vi "MM.vi"(0 "AppInst":refnum<vi>, 1 "ActorMethod":path, 2 "ActorClassItemRef(Don't Delete)":refnum<vi>, 3 "OnlyUpdate(if needed,False)":bool, 4 "Destination Path":path, 5 "error in":errorcluster, 6 "TemplatePath":path, 8 "TemplateVersion":string) -> (19 "error out":errorcluster)   [LabVIEW 2020]
uses:
  <vilib>/Utility/VariantDataType/Type.ctl
  <vilib>/Utility/miscctls.llb/LVPositionTypeDef.ctl
  <vilib>/Utility/traverseref.llb/TRef TravTarget.ctl
  <resource>/Framework/Providers/Open_GDS/ClassProviders/Common/LvClass_class/GDSLvCLass_ClassSettingsType.ctl
  <resource>/Framework/Providers/Open_GDS/ClassProviders/Common/LvClass_class/GDSLvClass_PlugIn.ctl
  <resource>/Framework/Providers/Open_GDS/ClassProviders/Common/LvClass_class/GDSLvClass_PlugInTypes.ctl
  <resource>/Framework/Providers/Open_GDS/ClassProviders/Provider_LvNativeClass/LvNativeProviderName.ctl
  <vilib>/Utility/VariantDataType/VariantType.lvlib
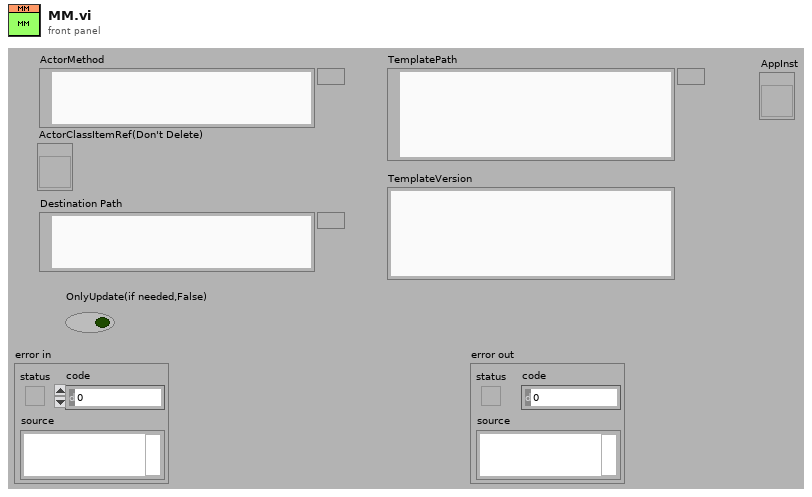
[diagram p1: front panel]
types:
  T1 = cluster{"Counter":i32, "DebugInfo":string, "Update":bool, "Target Actor Method path":path, "Class Name":string, "New Class Path":path, "Wiring Rules":enum16{"Invalid Wire Rule", "Required", "Recommended", "Optional", "Dynamic Dispatch"}[], "New Send Method":path, "Pattern":u32, "NewClassName":string, "NewClasstypeString":string, "Destination Path":path, "MessageClassRef":refnum<vi>, "Version":string, "ActorClassRef":refnum<vi>, "QualifiedNameOfLibrary":string, "TemplatePath":path, "ActorClassPath":path, "MemberDataTypes":cluster{"Label.Text":string, "Style":u32}[], "MemberData":refnum<vi>, "ActorClassParentItem":refnum<vi>}
  T2 = enum32{"Invalid", "Standard", "Closed", "Hidden", "Minimized", "Maximized"}
  T3 = typedef "LVPositionTypeDef.ctl" = cluster{"Left":i32, "Top":i32}
  T4 = typedef "TRef TravTarget.ctl" = enum16{"FP", "BD", "Other"}
  T5 = typedef "LvNativeProviderName.ctl" = enum16{"Endevo LabVIEW Native"}
  T6 = typedef "GDSLvCLass_ClassSettingsType.ctl" = cluster{"ClassProviderName":string, "ClassTemplateUsed":string, "ClassTemplateVersion":string, "ClassDescription":string, "PlugIns":T7[], "ConnectorPanePattern":string}
  T7 = typedef "GDSLvClass_PlugIn.ctl" = cluster{"Type":T8, "ID":string, "Version":string, "Path":path, "Name":string, "Data":variant}
  T8 = typedef "GDSLvClass_PlugInTypes.ctl" = enum16{"DesignPattern", "MethodTypes"}
  T9 = cluster{"LibraryIcon":string, "HeaderRows(1)":u8}
  T10 = enum32{"invalid VI type", "Standard VI", "Control VI", "Global VI", "Polymorphic VI", "Configuration VI", "SubSystem", "Facade VI", "Method VI", "Statechart Diagram VI"}
  T11 = typedef "AF_SettingsType.ctl" = cluster{"MessageFolderName":string}
  T12 = cluster{"Major":u16, "Minor":u16, "Fix":u16, "Build":u16}
  T13 = typedef "GOOP_WireConfigurationType.ctl" = cluster{"Edge thickness":i32, "Edge color":u32, "Center thickness":i32, "Center pattern":T14, "CenterColor1":u32, "CenterColor2":u32, "Tunnels and terminals colors":u32}
  T14 = typedef "GOOP_WirePattern.ctl" = enum16{"Solid", "Large dash", "Small dash"}
  T15 = cluster{"Foreground Color":u32, "Background Color":u32, "Fill Pattern":cluster{"Row 0":u8, "Row 1":u8, "Row 2":u8, "Row 3":u8, "Row 4":u8, "Row 5":u8, "Row 6":u8, "Row 7":u8}, "Width":i16, "Mode":enum16{"Copy", "Or", "Exclusive Or", "Bit Clear", "Not Copy", "Not Or", "Nor Exclusive Or", "Not Bit Clear"}, "Style":enum32{"Solid", "Dash", "Dot", "Dash Dot", "Dash Dot Dot"}, "Fill Rule":enum32{"Even Odd", "Winding"}, "End Caps":enum32{"Default", "Flat"}}[]
  T16 = enum16{"Invalid Wire Rule", "Required", "Recommended", "Optional", "Dynamic Dispatch"}[]
  T17 = typedef "VariantType.lvlib/Type.ctl" = enum8{"Invalid Type", "Void", "I8", "I16", "I32", "I64", "U8", "U16", "U32", "U64", "Single Float", "Double Float", "Extended Float", "Single Complex", "Double Complex", "Extended Complex", "Enum U8", "Enum U16", "Enum U32", "Enum U64", "Single Float With Unit", "Double Float With Unit", "Extended Float With Unit", "Single Complex with Unit", "Double Complex with Unit", "Extended Complex with Unit", "Boolean", "String", "Path", "Picture", "Tag", "Array", "Cluster", "Variant", "LV Variant", "Waveform", "Timestamp", "Digital Waveform", "Digital Data", "ExpressData", "Refnum", "External Data", "VI", "Poly VI", "LabVIEW Class Instance", "Fixed Point"}
  T18 = typedef "LVRectTypeDef.ctl" = cluster{"Left":i16, "Top":i16, "Right":i16, "Bottom":i16}
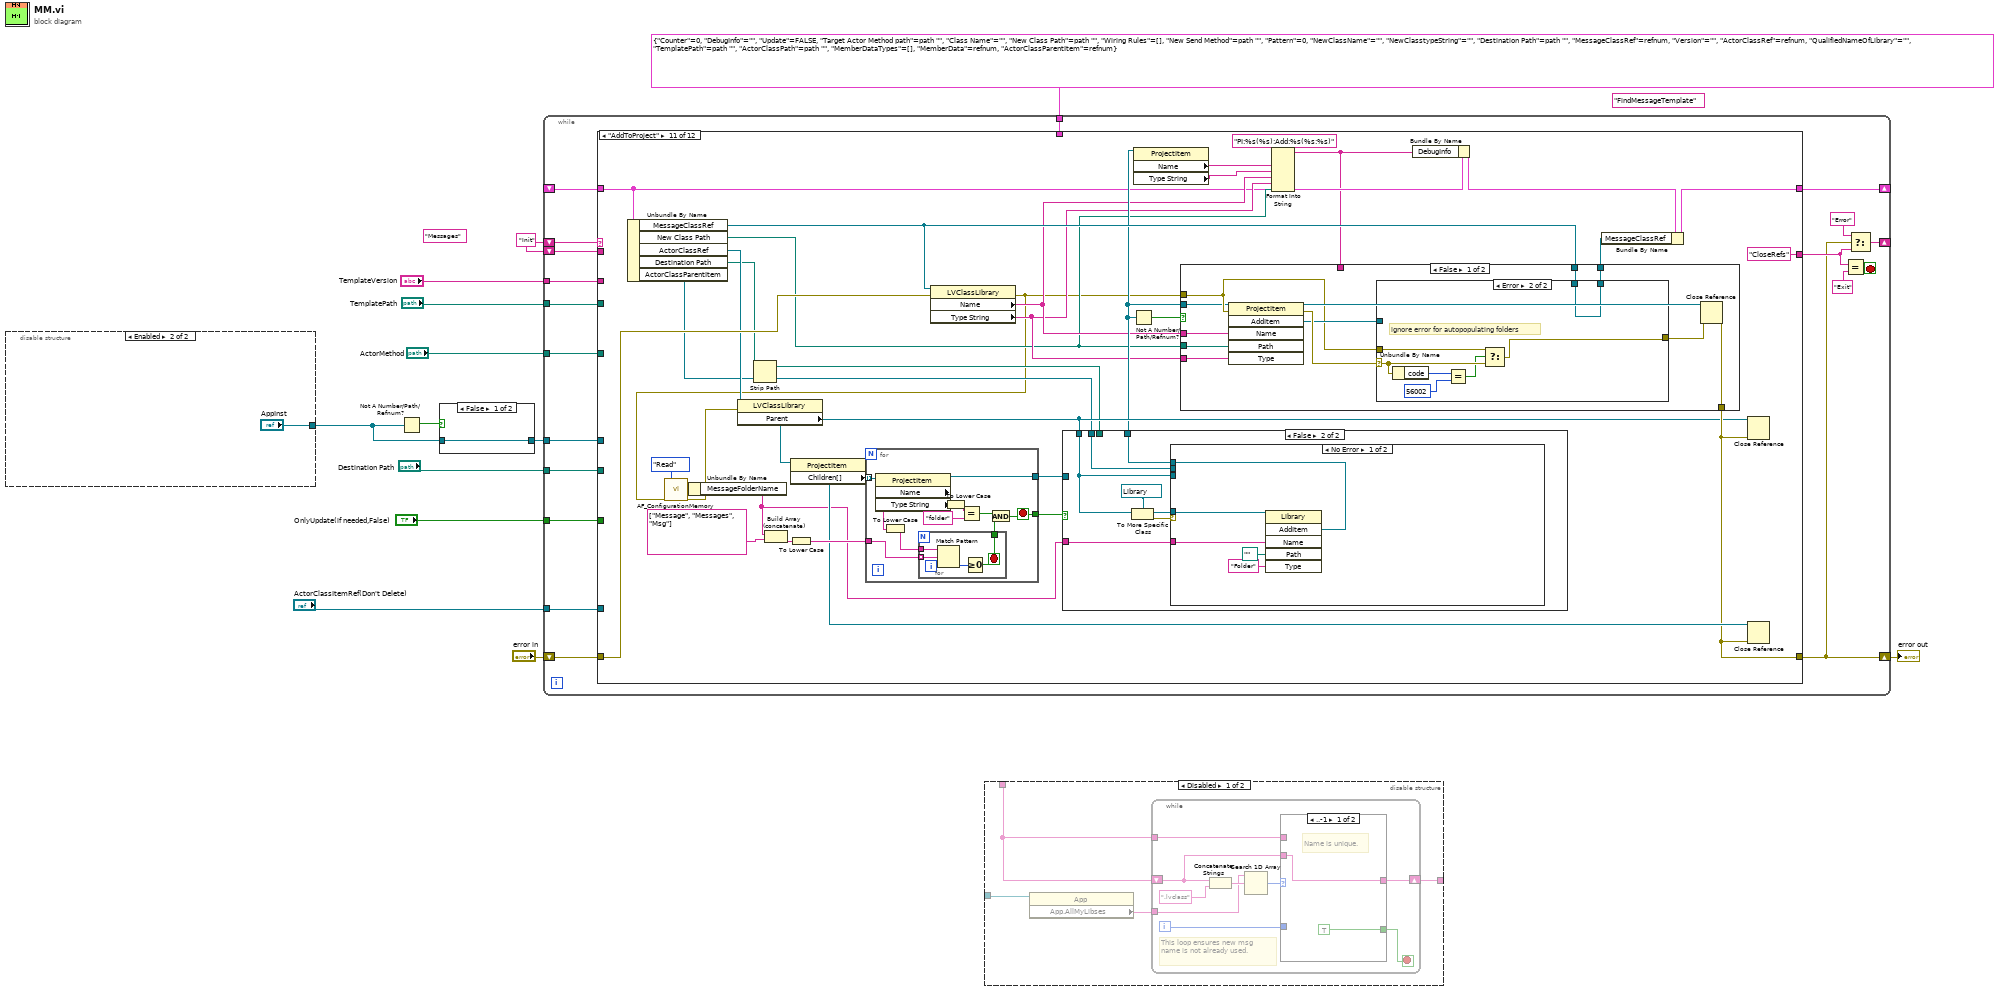
[diagram p0: block diagram]
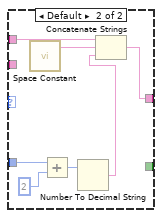
[diagram p2: hidden frame]
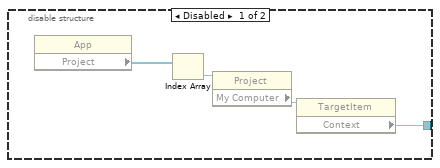
[diagram p4: hidden frame]
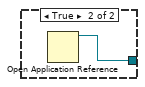
[diagram p5: hidden frame]
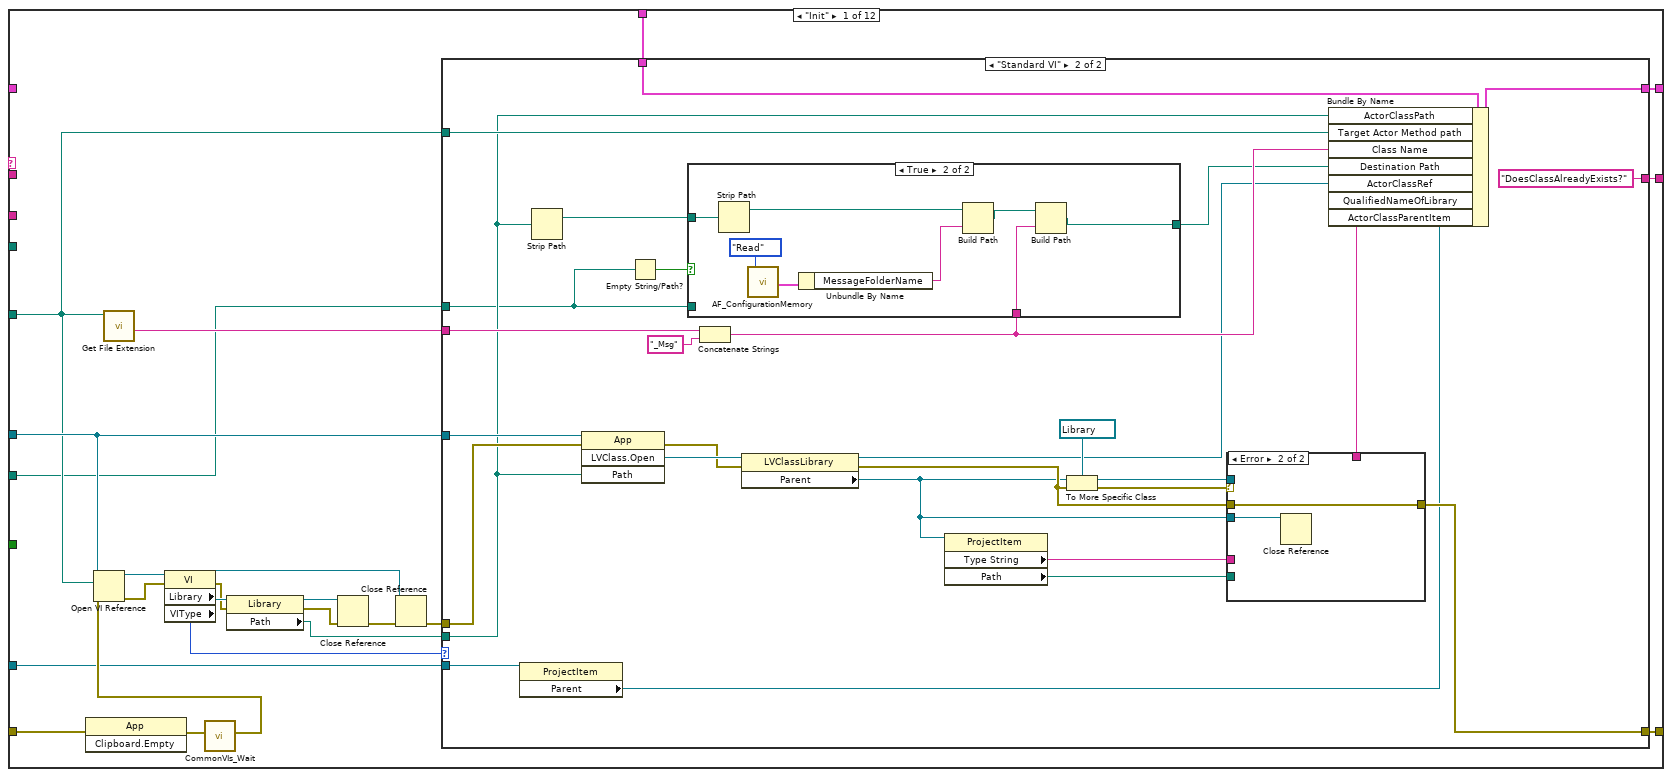
[diagram p6: hidden frame]
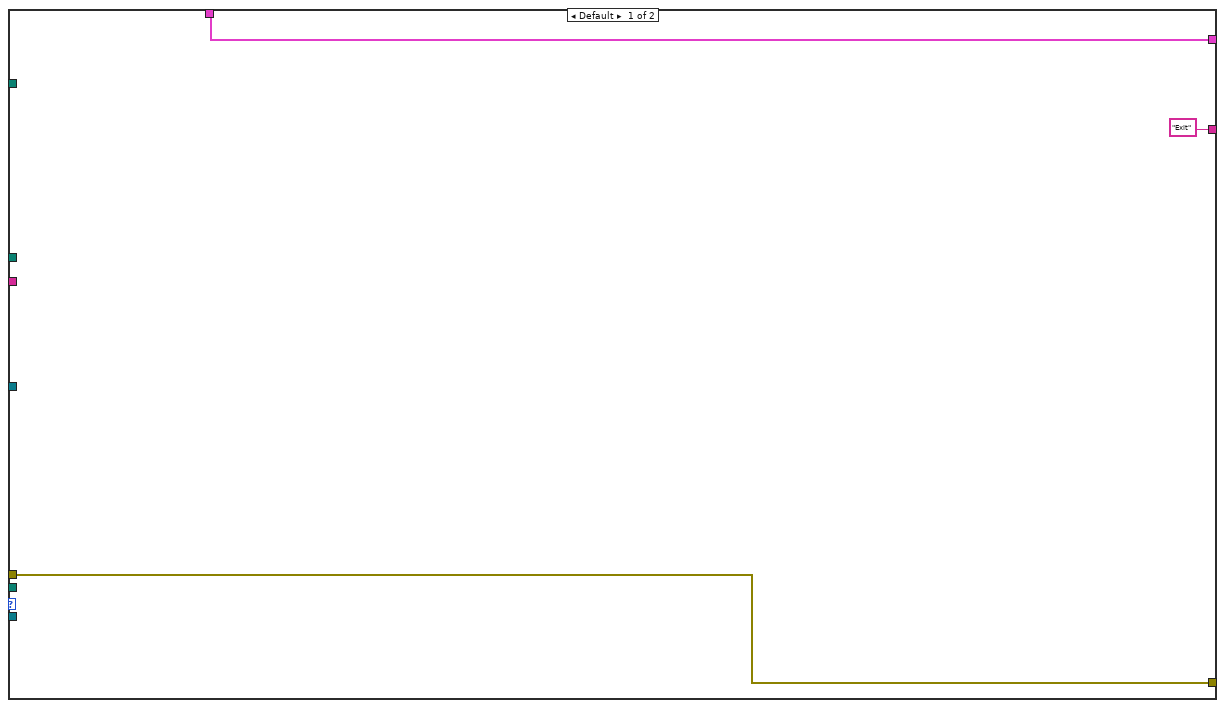
[diagram p7: hidden frame]
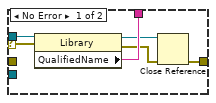
[diagram p8: hidden frame]
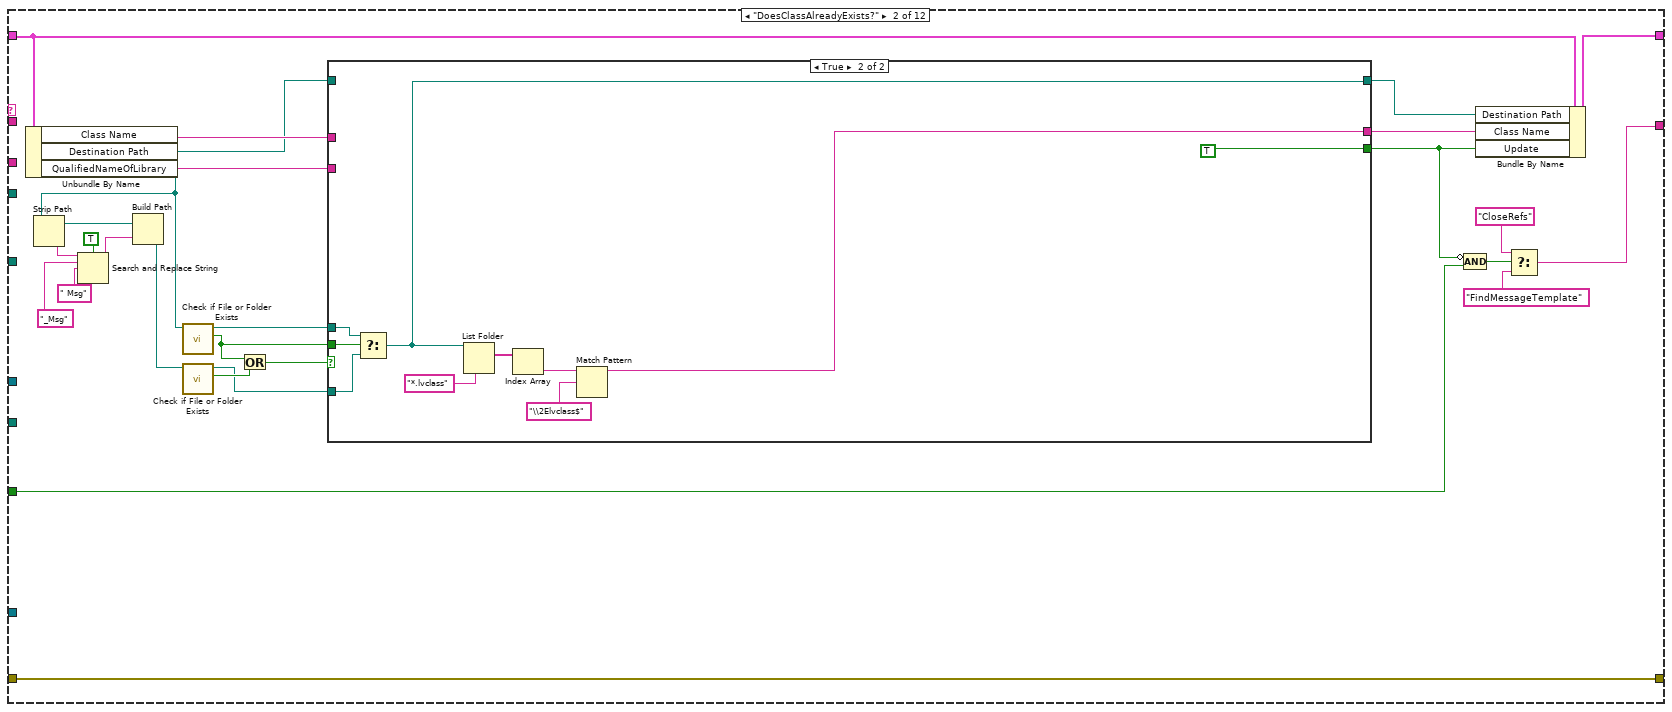
[diagram p10: hidden frame]
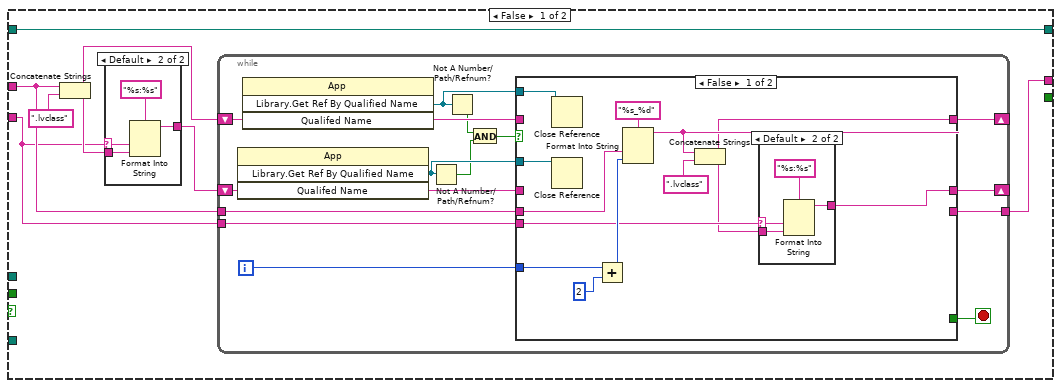
[diagram p11: hidden frame]
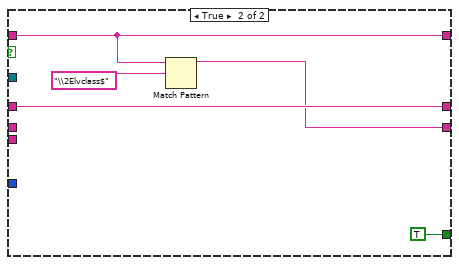
[diagram p13: hidden frame]
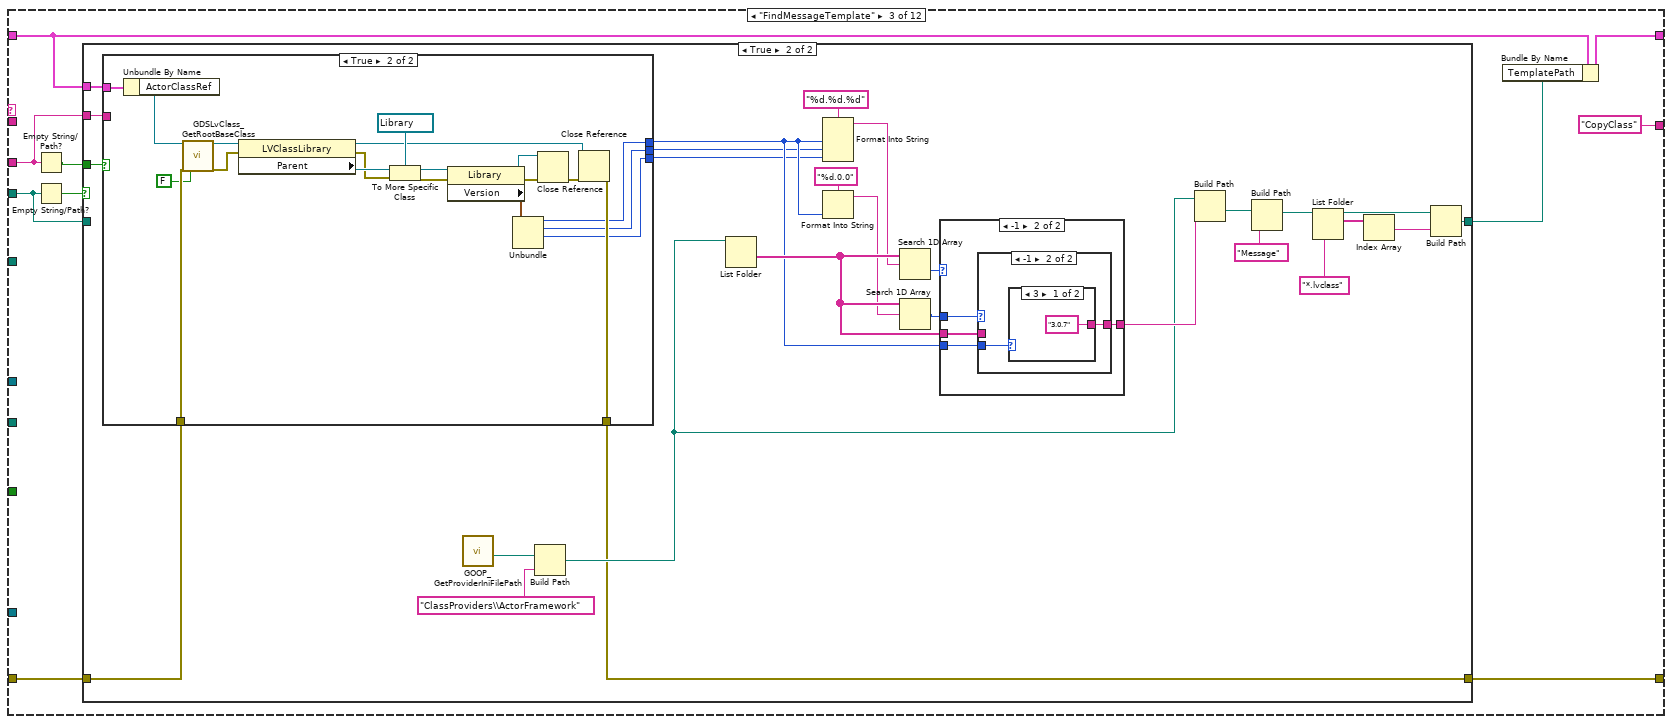
[diagram p15: hidden frame]
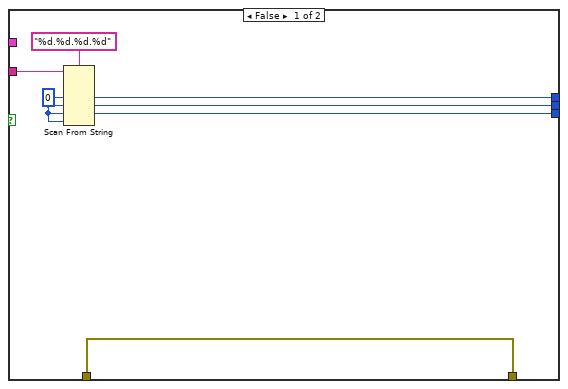
[diagram p17: hidden frame]
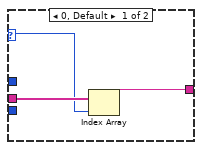
[diagram p18: hidden frame]
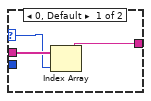
[diagram p19: hidden frame]
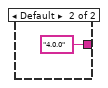
[diagram p20: hidden frame]
diagram:
  (unwired) "FindMessageTemplate"
  (unwired) "Messages" ("Name")
  w1 = "Init"
  n1 = disable-structure shown="Enabled" {
    disable-tunnel: [w14 "AppInst"] -> w4
    frame Disabled {
      n2 = property class="App"() -> ("Project"=w17:refnum<vi>[])  [unwired: 2 in, 2 out]
      n3 = Index Array(array=w17) -> (element=w16:refnum<vi>)  [unwired: 1 in]
      n4 = property class="Project"(reference=w16) -> ("My Computer"=w15:refnum<vi>)  [unwired: 1 in, 2 out]
      n5 = property class="TargetItem"(reference=w15) -> ("Context"=w14:refnum<vi>)  [unwired: 1 in, 2 out]
    }
    frame Enabled {
    }
  }
  n6 = Not A Number/Path/Refnum?(number/path/refnum=w4) -> (NaN/Path/Refnum?=w8:bool)
  n7 = case shown="False" w8 {
    tunnel: [w19 w20] -> w7
    tunnel: w4 -> [w19 _]
    frame False {
    }
    frame True {
      n8 = Open Application Reference() -> (3:w20:refnum<vi>)  [unwired: 4 in, 1 out]
    }
  }
  n9 = while {
    shift-right: [w25] -> w12
    shift-left: "error in" -> [w39]
    shift-right: [w37] -> _
    shift-left: w1 -> [w38]
    shift-right: [w32] -> _
    shift-left: _ -> [w31]
    tunnel: "ActorMethod" -> [w30]
    tunnel: T1 {"Counter"=0, "DebugInfo"="", "Update"=FALSE, "Target Actor Method path"=path "", "Class Name"="", "New Class Path"=path "", "Wiring Rules"=[], "New Send Method"=path "", "Pattern"=0, "NewClassName"="", "NewClasstypeString"="", "Destination Path"=path "", "MessageClassRef"=refnum, "Version"="", "ActorClassRef"=refnum, "QualifiedNameOfLibrary"="", "TemplatePath"=path "", "ActorClassPath"=path "", "MemberDataTypes"=[], "MemberData"=refnum, "ActorClassParentItem"=refnum} -> [w29]
    tunnel: "Destination Path" -> [w28]
    tunnel: "TemplatePath" -> [w27]
    tunnel: w7 -> [w26]
    tunnel: "TemplateVersion" -> [w24]
    tunnel: "OnlyUpdate(if needed,False)" -> [w23]
    tunnel: "ActorClassItemRef(Don't Delete)" -> [w22]
    shift-left: w1 -> [w21]
    stop <- w36 stop-if-true
    n10 = case shown="\"AddToProject\"" w38 {
      tunnel: w39 -> [w42 w132 w196 w280 w381 w503 w601 w665 w739 w831 w903 w983]
      tunnel: [w62 w124 "CopyClass" "CopyMemberData" "AddMemberData" w495 "BuildSendMethod" "BuildDo" w711 "AddToProject" "CloseRefs" "Exit"] -> w33
      tunnel: [w61 w131 w204 w290 w376 w488 w597 w661 w708 w837 w902 w970] -> w32
      tunnel: w31 -> [_ w134 w197 w291 w378 w489 w598 w661 w708 w837 w876 w970]
      tunnel: w30 -> [w52 _ _ _ _ _ w590 _ _ w827 _ _]
      tunnel: w29 -> [w45 _ _ _ _ _ _ _ _ _ _ _]
      tunnel: w28 -> [w50 _ _ _ _ _ _ _ _ _ _ _]
      tunnel: w27 -> [_ _ w199 _ _ _ _ _ _ w834 _ _]
      tunnel: w26 -> [w59 _ _ w277 w380 _ w600 w663 w740 _ _ w980]
      tunnel: [w60 w132 w195 w285 w379 w490 w602 w664 w737 w835 w894 w972] -> w25
      tunnel: w24 -> [_ _ w202 _ _ _ _ _ _ _ _ _]
      tunnel: w23 -> [_ w129 _ _ _ _ _ _ _ _ _ _]
      tunnel: w22 -> [w40 _ _ _ _ _ _ _ _ _ _ _]
      tunnel: w21 -> [_ _ _ _ _ _ _ _ _ _ _ w971]
      frame "Init" {
        n11 = invoke class="App" method="Clipboard.Empty"(error in=w42) -> (error out=w43:errorcluster)  [unwired: 2 in, 2 out]
        n12 = call <vilib>:"Get File Extension.vi"("file"=w52) -> ("filename without extension"=w51:string)  [unwired: 6 in, 4 out]
        n13 = call <resource>:"CommonVIs_Wait.vi"("error in"=w43) -> ("error out"=w41:errorcluster)  [unwired: 9 in]
        n14 = Open VI Reference(application reference (local)=w59, vi path=w52, error in (no error)=w41) -> (vi reference=w58:refnum<vi>, error out=w57:errorcluster)  [unwired: 3 in]
        n15 = property class="VI"(reference=w58, error in=w57) -> (reference out=w48:refnum<vi>, error out=w53:errorcluster, "Library"=w56:refnum<vi>, "VIType"=w44:T10)
        n16 = property class="Library"(reference=w56, error in=w53) -> (reference out=w55:refnum<vi>, error out=w54:errorcluster, "Path"=w46:path)
        n17 = Close Reference(reference=w55, error in (no error)=w54) -> (error out=w49:errorcluster)
        n18 = Close Reference(reference=w48, error in (no error)=w49) -> (error out=w47:errorcluster)
        n19 = case shown="\"Standard VI\"" w44 {
          tunnel: ["Exit" "DoesClassAlreadyExists?"] -> w62
          tunnel: [w64 w92] -> w61
          tunnel: [w63 w81] -> w60
          tunnel: w59 -> [_ w80]
          tunnel: w52 -> [_ w79]
          tunnel: w51 -> [_ w78]
          tunnel: w50 -> [_ w72]
          tunnel: w47 -> [w63 w77]
          tunnel: w46 -> [_ w73]
          tunnel: w45 -> [w64 w76]
          tunnel: w40 -> [_ w67]
          frame Default {
          }
          frame "Standard VI" {
            n20 = property class="ProjectItem"(reference=w67) -> ("Parent"=w66:refnum<vi>)  [unwired: 1 in, 2 out]
            n21 = Strip Path(path=w73) -> (stripped path=w90:path)  [unwired: 1 out]
            n22 = invoke class="App" method="LVClass.Open"(reference=w80, error in=w77, "Path"=w73) -> (error out=w74:errorcluster, "LVClass.Open"=w75:refnum<vi>)  [unwired: 1 in, 2 out]
            n23 = Empty String/Path?(string/path=w72) -> (empty?=w88:bool)
            n24 = Concatenate Strings(w78, "_Msg" ("string")) -> (w89:string)
            n25 = case shown="True" w88 {
              tunnel: w72 -> [w102 _]
              tunnel: [w102 w106] -> w71
              tunnel: w90 -> [_ w110]
              tunnel: w89 -> [_ w107]
              frame False {
              }
              frame True {
                n26 = Strip Path(path=w110) -> (stripped path=w109:path)  [unwired: 1 out]
                n27 = call <resource>:"AF_ConfigurationMemory.vi"("Action"=enum16{"Read", "Load", "Save", "Set"}."Read") -> ("AF_SettingsOut"=w104:T11)  [unwired: 15 in, 3 out]
                n28 = Unbundle By Name(w104) -> ("MessageFolderName"=w103:string)
                n29 = Build Path(base path=w109, name or relative path=w103) -> (appended path=w108:path)
                n30 = Build Path(base path=w108, name or relative path=w107) -> (appended path=w106:path)
              }
            }
            n31 = property class="LVClassLibrary"(reference=w75, error in=w74) -> (reference out=w83:refnum<vi>, error out=w84:errorcluster, "Parent"=w70:refnum<vi>)
            n32 = property class="ProjectItem"(reference=w70) -> ("Type String"=w69:string, "Path"=w68:path)  [unwired: 1 in, 2 out]
            n33 = To More Specific Class(target class=refnum<vi> refnum ("reference out"), reference=w70, error in=w84) -> (specific class reference=w86:refnum<vi>, error out=w85:errorcluster)
            n34 = case shown="Error" w85 {
              selector: w85 -> [w98 _]
              tunnel: w86 -> [w99 _]
              tunnel: w84 -> [_ w101]
              tunnel: [w97 _] -> w82
              tunnel: [w94 w101] -> w81
              tunnel: w70 -> [_ w100]
              tunnel: w69 -> [_ _]
              tunnel: w68 -> [_ _]
              frame No Error {
                n35 = property class="Library"(reference=w99, error in=w98) -> (reference out=w96:refnum<vi>, error out=w95:errorcluster, "QualifiedName"=w97:string)
                n36 = Close Reference(reference=w96, error in (no error)=w95) -> (error out=w94:errorcluster)
              }
              frame Error {
                n37 = Close Reference(reference=w100) -> ()  [unwired: 1 in, 1 out]
              }
            }
            n38 = Bundle By Name(cluster=w76, "ActorClassPath"=w73, "Target Actor Method path"=w79, "Class Name"=w89, "Destination Path"=w71, "ActorClassRef"=w83, "QualifiedNameOfLibrary"=w82, "ActorClassParentItem"=w66) -> (w92:T1)
          }
        }
      }
      frame "DoesClassAlreadyExists?" {
        n39 = Unbundle By Name(w134) -> ("Class Name"=w136:string, "Destination Path"=w112:path, "QualifiedNameOfLibrary"=w135:string)
        n40 = Strip Path(path=w112) -> (stripped path=w123:path, name=w122:string)
        n41 = Search and Replace String(case sensitive?=TRUE ("ignore case? (F)"), input string=w122, search string="_Msg" ("string"), replace string=" Msg" ("string")) -> (result string=w118:string)  [unwired: 4 in, 3 out]
        n42 = Build Path(base path=w123, name or relative path=w118) -> (appended path=w116:path)
        n43 = call <vilib>:"Check if File or Folder Exists.vi"("path"=w112) -> ("file or folder exists?"=w114:bool, "dup path"=w130:path)  [unwired: 8 in, 1 out]
        n44 = call <vilib>:"Check if File or Folder Exists.vi"("path"=w116) -> ("file or folder exists?"=w117:bool, "dup path"=w113:path)  [unwired: 8 in, 1 out]
        n45 = Or(x=w114, y=w117) -> (x .or. y?=w115:bool)
        n46 = case shown="True" w115 {
          tunnel: w136 -> [w142 _]
          tunnel: w135 -> [w138 _]
          tunnel: [w139 w189] -> w133
          tunnel: [_ TRUE] -> w128
          tunnel: w130 -> [_ w186]
          tunnel: w114 -> [_ w188]
          tunnel: w113 -> [_ w187]
          tunnel: w112 -> [w137 _]
          tunnel: [w137 w185] -> w111
          frame False {
            n47 = Concatenate Strings(w142, ".lvclass" ("regular expression")) -> (w140:string)
            n48 = case shown="Default" w138 {
              selector: w138 -> [_ w181]
              tunnel: w140 -> [w180 w183]
              tunnel: [w180 w182] -> w141
              frame "" {
              }
              frame Default {
                n49 = Format Into String(format string="%s:%s", w181, w183) -> (resulting string=w182:string)  [unwired: 2 in, 1 out]
              }
            }
            n50 = while {
              shift-right: [w153] -> _
              shift-left: w141 -> [w151]
              tunnel: w142 -> [w156]
              tunnel: w138 -> [w155]
              tunnel: [w150] -> w139
              shift-right: [w149] -> _
              shift-left: w140 -> [w148]
              i -> [w157]
              stop <- w152 stop-if-true
              n51 = invoke class="App" method="Library.Get Ref By Qualified Name"("Qualifed Name"=w151) -> ("Library.Get Ref By Qualified Name"=w154:refnum<vi>)  [unwired: 3 in, 3 out]
              n52 = invoke class="App" method="Library.Get Ref By Qualified Name"("Qualifed Name"=w148) -> ("Library.Get Ref By Qualified Name"=w144:refnum<vi>)  [unwired: 3 in, 3 out]
              n53 = Not A Number/Path/Refnum?(number/path/refnum=w154) -> (NaN/Path/Refnum?=w146:bool)
              n54 = Not A Number/Path/Refnum?(number/path/refnum=w144) -> (NaN/Path/Refnum?=w147:bool)
              n55 = And(x=w147, y=w146) -> (x .and. y?=w145:bool)
              n56 = case shown="False" w145 {
                tunnel: w157 -> [w168 _]
                tunnel: w156 -> [w166 _]
                tunnel: w155 -> [w163 _]
                tunnel: w154 -> [w162 _]
                tunnel: [w161 w178] -> w153
                tunnel: [_ TRUE] -> w152
                tunnel: w151 -> [_ w178]
                tunnel: [w160 w175] -> w150
                tunnel: [w159 w177] -> w149
                tunnel: w148 -> [_ w177]
                tunnel: w144 -> [w158 _]
                frame False {
                  n57 = Close Reference(reference=w158) -> ()  [unwired: 1 in, 1 out]
                  n58 = Close Reference(reference=w162) -> ()  [unwired: 1 in, 1 out]
                  n59 = Add(x=w168, y=2) -> (x+y=w164:i32)
                  n60 = Format Into String(format string="%s_%d", w166, w164) -> (resulting string=w160:string)  [unwired: 2 in, 1 out]
                  n61 = Concatenate Strings(w160, ".lvclass" ("regular expression")) -> (w159:string)
                  n62 = case shown="Default" w163 {
                    selector: w163 -> [_ w171]
                    tunnel: w159 -> [w170 w173]
                    tunnel: [w170 w172] -> w161
                    frame "" {
                    }
                    frame Default {
                      n63 = Format Into String(format string="%s:%s", w171, w173) -> (resulting string=w172:string)  [unwired: 2 in, 1 out]
                    }
                  }
                }
                frame True {
                  n64 = Match Pattern(string=w177, regular expression="\\2Elvclass$") -> (before substring=w175:string)  [unwired: 1 in, 3 out]
                }
              }
            }
          }
          frame True {
            n65 = Select(t=w186, s=w188, f=w187) -> (s? t:f=w185:path)
            n66 = List Folder(path=w185, pattern="*.lvclass") -> (filenames=w191:string[])  [unwired: 2 in, 3 out]
            n67 = Index Array(array=w191) -> (element=w190:string)  [unwired: 1 in]
            n68 = Match Pattern(string=w190, regular expression="\\2Elvclass$") -> (before substring=w189:string)  [unwired: 1 in, 3 out]
          }
        }
        n69 = Compound Arithmetic op=AND(invert w128, w129) -> (w127:bool)
        n70 = Bundle By Name(cluster=w134, "Destination Path"=w111, "Class Name"=w133, "Update"=w128) -> (w131:T1)
        n71 = Select(t="CloseRefs", s=w127, f="FindMessageTemplate") -> (s? t:f=w124:string)
      }
      frame "FindMessageTemplate" {
        n72 = Empty String/Path?(string/path=w202) -> (empty?=w198:bool)
        n73 = Empty String/Path?(string/path=w199) -> (empty?=w200:bool)
        n74 = case shown="True" w200 {
          tunnel: w202 -> [_ w231]
          tunnel: [w206 w224] -> w201
          tunnel: w199 -> [w206 _]
          tunnel: w198 -> [_ w212]
          tunnel: w197 -> [_ w210]
          tunnel: w196 -> [w205 w209]
          tunnel: [w205 w208] -> w195
          frame False {
          }
          frame True {
            n75 = case shown="True" w212 {
              tunnel: w231 -> [w240 _]
              tunnel: [w238 w244] -> w215
              tunnel: [w237 w243] -> w214
              tunnel: [w236 w242] -> w213
              tunnel: w210 -> [_ w253]
              tunnel: w209 -> [w235 w251]
              tunnel: [w235 w246] -> w208
              frame False {
                w234 = u16 0 ("default value 1")
                n76 = Scan From String(format string="%d.%d.%d.%d", input string=w240, default 1=w234, default 2=w234, default 3=w234, default 4=w234) -> (output 1=w238:u16, output 2=w237:u16, output 3=w236:u16)  [unwired: 3 in, 3 out]
              }
              frame True {
                n77 = Unbundle By Name(w253) -> ("ActorClassRef"=w252:refnum<vi>)
                n78 = call <resource>:"GDSLvClass_GetRootBaseClass.vi"("ViRef/Path,LvClassRef/Path"=w252, "error in (no error)"=w251, "LimitToSpecificProviderTypeOfSameType(True)"=FALSE) -> ("RootBaseClassRef"=w260:refnum<vi>, "error out"=w258:errorcluster)  [unwired: 11 in, 4 out]
                n79 = property class="LVClassLibrary"(reference=w260, error in=w258) -> (reference out=w247:refnum<vi>, error out=w256:errorcluster, "Parent"=w257:refnum<vi>)
                n80 = To More Specific Class(target class=refnum<vi> refnum ("reference out"), reference=w257, error in=w256) -> (specific class reference=w255:refnum<vi>, error out=w254:errorcluster)
                n81 = property class="Library"(reference=w255, error in=w254) -> (reference out=w249:refnum<vi>, error out=w250:errorcluster, "Version"=w245:T12)
                n82 = Unbundle(w245) -> ("Major"=w244:u16, "Minor"=w243:u16, "Fix"=w242:u16)  [unwired: 1 out]
                n83 = Close Reference(reference=w249, error in (no error)=w250) -> (error out=w248:errorcluster)
                n84 = Close Reference(reference=w247, error in (no error)=w248) -> (error out=w246:errorcluster)
              }
            }
            n85 = call <resource>:"GOOP_GetProviderIniFilePath.vi"() -> ("ProviderMainFolder"=w233:path)  [unwired: 10 in, 1 out]
            n86 = Build Path(base path=w233, name or relative path="ClassProviders\\ActorFramework") -> (appended path=w211:path)
            n87 = List Folder(path=w211) -> (folder names=w222:string[])  [unwired: 3 in, 3 out]
            n88 = Format Into String(format string="%d.%d.%d", w215, w214, w213) -> (resulting string=w218:string)  [unwired: 2 in, 1 out]
            n89 = Format Into String(format string="%d.0.0", w215) -> (resulting string=w219:string)  [unwired: 2 in, 1 out]
            n90 = Search 1D Array(1D array=w222, element=w218) -> (index of element=w220:i32)  [unwired: 1 in]
            n91 = Search 1D Array(1D array=w222, element=w219) -> (index of element=w221:i32)  [unwired: 1 in]
            n92 = case shown="-1" w220 {
              selector: w220 -> [w262 _]
              tunnel: w221 -> [_ w267]
              tunnel: [w261 w266] -> w223
              tunnel: w222 -> [w263 w265]
              tunnel: w215 -> [_ w264]
              frame 0, Default {
                n93 = Index Array(array=w263, index=w262) -> (element=w261:string)
              }
              frame -1 {
                n94 = case shown="-1" w267 {
                  selector: w267 -> [w269 _]
                  tunnel: [w268 w272] -> w266
                  tunnel: w265 -> [w270 _]
                  tunnel: w264 -> [_ w271]
                  frame 0, Default {
                    n95 = Index Array(array=w270, index=w269) -> (element=w268:string)
                  }
                  frame -1 {
                    n96 = case shown="3" w271 {
                      tunnel: ["3.0.7" ("TemplateIdName") "4.0.0" ("TemplateIdName")] -> w272
                      frame 3 {
                      }
                      frame Default {
                      }
                    }
                  }
                }
              }
            }
            n97 = Build Path(base path=w211, name or relative path=w223) -> (appended path=w229:path)
            n98 = Build Path(base path=w229, name or relative path="Message") -> (appended path=w207:path)
            n99 = List Folder(path=w207, pattern="*.lvclass") -> (path out=w225:path, filenames=w227:string[])  [unwired: 2 in, 2 out]
            n100 = Index Array(array=w227) -> (element=w226:string)  [unwired: 1 in]
            n101 = Build Path(base path=w225, name or relative path=w226) -> (appended path=w224:path)
          }
        }
        n102 = Bundle By Name(cluster=w197, "TemplatePath"=w201) -> (w204:T1)
      }
      frame "CopyClass" {
        n103 = Unbundle By Name(w291) -> ("Class Name"=w282:string, "Destination Path"=w281:path, "Update"=w279:bool, "TemplatePath"=w278:path)
        n104 = case shown="False" w279 {
          tunnel: w278 -> [w326 _]
          tunnel: [w292 w330] -> w288
          tunnel: [w325 _] -> w287
          tunnel: [w293 w329] -> w275
          tunnel: w282 -> [w324 w334]
          tunnel: w281 -> [w297 w332]
          tunnel: w280 -> [w316 w331]
          tunnel: w277 -> [w299 w327]
          tunnel: [w294 w328] -> w276
          frame False {
            n105 = call <resource>:"File_CreateFolders.vi"("Path"=w297, "error in (no error)"=w316) -> ("error out"=w315:errorcluster)  [unwired: 15 in, 2 out]
            n106 = invoke class="App" method="LVClass.Open"(error in=w315, "Path"=w326) -> (error out=w305:errorcluster, "LVClass.Open"=w314:refnum<vi>)  [unwired: 2 in, 2 out]
            n107 = Concatenate Strings(w324, ".lvclass" ("regular expression")) -> (w295:string)
            n108 = property class="LVClassLibrary"(reference=w314, error in=w305) -> (reference out=w304:refnum<vi>, error out=w303:errorcluster, "Version"=w317:T12)
            n109 = invoke class="LVClassLibrary" method="Save a Copy"(reference=w304, error in=w303, "Path"=w297, "New Name"=w295) -> (reference out=w301:refnum<vi>, error out=w302:errorcluster, "New Lib Path"=w292:path)  [unwired: 2 in, 3 out]
            n110 = Close Reference(reference=w301, error in (no error)=w302) -> (error out=w300:errorcluster)
            n111 = invoke class="App" method="LVClass.Open"(reference=w299, error in=w300, "Path"=w292) -> (error out=w298:errorcluster, "LVClass.Open"=w296:refnum<vi>)  [unwired: 1 in, 2 out]
            n112 = call <resource>:"AF_ConfigurationMemory.vi"("error in (no error)"=w298, "Action"=enum16{"Read", "Load", "Save", "Set"}."Read") -> ("AF_MessaageWireConfigurationOut"=w311:T13, "IconOut"=w312:string, "error out"=w313:errorcluster)  [unwired: 14 in, 1 out]
            n113 = call <resource>:"GOOP_WirePenTranslator.vi"("WireConfigurationIn"=w311) -> ("WirePensOut"=w309:T15)  [unwired: 17 in, 1 out]
            n114 = call <resource>:"GDSLvClass_StoreClassItemIcon.vi"("Library Refnum"=w296, "ClassItemIconName"=w312, "error in (no error)"=w313) -> ("error out"=w308:errorcluster)  [unwired: 15 in, 1 out]
            n115 = property class="LVClassLibrary"(reference=w296, error in=w308, "Wire Pens"=w309) -> (reference out=w307:refnum<vi>, error out=w306:errorcluster)
            n116 = Unbundle(w317) -> ("Major"=w321:u16, "Minor"=w320:u16, "Fix"=w319:u16, "Build"=w318:u16)
            n117 = invoke class="LVClassLibrary" method="Save"(reference=w307, error in=w306) -> (reference out=w294:refnum<vi>, error out=w293:errorcluster)  [unwired: 2 in, 2 out]
            n118 = Format Into String(format string="%d.%d.%d.%d", w321, w320, w319, w318) -> (resulting string=w325:string)  [unwired: 2 in, 1 out]
          }
          frame True {
            n119 = Concatenate Strings(w334, ".lvclass" ("regular expression")) -> (w333:string)
            n120 = Build Path(base path=w332, name or relative path=w333) -> (appended path=w330:path)
            n121 = invoke class="App" method="LVClass.Open"(reference=w327, error in=w331, "Path"=w330) -> (error out=w329:errorcluster, "LVClass.Open"=w328:refnum<vi>)  [unwired: 1 in, 2 out]
          }
        }
        n122 = property class="LVClassLibrary"(reference=w276, error in=w275) -> (reference out=w286:refnum<vi>, error out=w285:errorcluster, "Name"=w284:string, "Type String"=w283:string)
        n123 = Bundle By Name(cluster=w291, "Version"=w287, "New Class Path"=w288, "NewClassName"=w284, "NewClasstypeString"=w283, "MessageClassRef"=w286) -> (w290:T1)
      }
      frame "CopyMemberData" {
        w369 = T16 [] items=["Invalid Wire Rule", "Required", "Recommended", "Optional", "Dynamic Dispatch"] ("WiringRules[]")
        w352 = T17[] [enum."Boolean", enum."I32", enum."String"] items=["Invalid Type", "Void", "I8", "I16", "I32", "I64", "U8", "U16", "U32", "U64", "Single Float", "Double Float", "Extended Float", "Single Complex", "Double Complex", "Extended Complex", "Enum U8", "Enum U16", "Enum U32", "Enum U64", "Single Float With Unit", "Double Float With Unit", "Extended Float With Unit", "Single Complex with Unit", "Double Complex with Unit", "Extended Complex with Unit", "Boolean", "String", "Path", "Picture", "Tag", "Array", "Cluster", "Variant", "LV Variant", "Waveform", "Timestamp", "Digital Waveform", "Digital Data", "ExpressData", "Refnum", "External Data", "VI", "Poly VI", "LabVIEW Class Instance", "Fixed Point"]
        n124 = Unbundle By Name(w378) -> ("Target Actor Method path"=w345:path)
        n125 = invoke class="App" method="Clipboard.Empty"(reference=w380, error in=w381) -> (reference out=w373:refnum<vi>, error out=w361:errorcluster)  [unwired: 1 in, 1 out]
        n126 = Open VI Reference(application reference (local)=w373, vi path=w345, error in (no error)=w361) -> (vi reference=w341:refnum<vi>, error out=w359:errorcluster)  [unwired: 3 in]
        n127 = disable-structure shown="Enabled" {
          disable-tunnel: w341 -> [w389 w390]
          disable-tunnel: [w388 _] -> _
          disable-tunnel: [w387 w390] -> w340
          frame Disabled {
            n128 = invoke class="VI" method="FP.Open"(reference=w389, "Activate"=TRUE ("Activate?"), "State"=T2."Standard") -> (reference out=w387:refnum<vi>, error out=w388:errorcluster)  [unwired: 2 in, 3 out]
          }
          frame Enabled {
          }
        }
        n129 = property class="VI"(reference=w340, error in=w359) -> (reference out=w382:refnum<vi>, error out=w350:errorcluster, "Panel"=w362:refnum<vi>, "Library"=w347:refnum<vi>, "ConPane"=w371:refnum<vi>)
        n130 = property class="Library"(reference=w347, error in=w350) -> (reference out=w348:refnum<vi>, error out=w349:errorcluster, "QualifiedName"=w351:string)
        n131 = Close Reference(reference=w348, error in (no error)=w349) -> (error out=w364:errorcluster)
        n132 = Spreadsheet String To Array(delimiter (Tab)=":", format string="%s", spreadsheet string=w351, array type (2D Dbl)=string[] []) -> (array=w353:string[])
        n133 = property class="ConPane"(reference=w371, error in=w364) -> (reference out=w367:refnum<vi>, error out=w366:errorcluster, "Ctrls[]"=w365:refnum<vi>[], "TermBnds[]"=w372:T18[], "WiringRules[]"=w370:T16, "Pattern"=w374:u32)
        n134 = Close Reference(reference=w367, error in (no error)=w366) -> (error out=w368:errorcluster)
        n135 = for {
          tunnel: w365 -> [w402] mode=indexing
          tunnel: string[] ["status", "code", "source"] -> [w409]
          tunnel: w352 -> [w408]
          tunnel: w353 -> [w407]
          shift-right: [w403] -> w360
          shift-left: w368 -> [w406]
          shift-right: [w404] -> w344
          shift-left: refnum<vi>[] [] ("Controls[]") -> [w405]
          shift-right: [w399] -> w377
          shift-left: w369 -> [w400]
          tunnel: w370 -> [w398] mode=indexing
          tunnel: w372 -> [w397] mode=indexing
          n136 = Not A Number/Path/Refnum?(number/path/refnum=w402) -> (NaN/Path/Refnum?=w401:bool)
          n137 = case shown="False" w401 {
            tunnel: w402 -> [w431 _]
            tunnel: w409 -> [w428 _]
            tunnel: w408 -> [w427 _]
            tunnel: w407 -> [w425 _]
            tunnel: w406 -> [w423 w485]
            tunnel: w405 -> [w418 w484]
            tunnel: [w417 w484] -> w404
            tunnel: [w416 w485] -> w403
            tunnel: w400 -> [w414 w483]
            tunnel: [w413 w483] -> w399
            tunnel: w398 -> [w412 _]
            tunnel: w397 -> [w411 _]
            frame False {
              n138 = property class="Ctl"(reference=w431, error in=w423) -> (reference out=w415:refnum<vi>, error out=w422:errorcluster, "Indicator"=w430:bool, "IsOnConPane"=w410:bool, "DefVal"=w420:variant)
              n139 = call <vilib>:"GetTypeInfo.vi"("error in (no error)"=w422, "Variant"=w420) -> ("error out"=w421:errorcluster, "Type Enum"=w429:T17)  [unwired: 5 in, 3 out]
              n140 = case shown="\"Cluster\"" w429 {
                tunnel: w420 -> [_ _ w465 w482]
                tunnel: w428 -> [_ _ w461 _]
                tunnel: w427 -> [_ _ w460 _]
                tunnel: [TRUE FALSE w457 w471] -> w426
                tunnel: w425 -> [_ _ _ w479]
                tunnel: w421 -> [w445 w447 w456 w481]
                tunnel: [w445 w447 w455 w480] -> w419
                tunnel: w411 -> [_ _ w454 w472]
                frame "Invalid Type", "Void" {
                }
                frame "I8", Default {
                }
                frame "Cluster" {
                  n141 = call <vilib>:"GetClusterInfo.vi"("error in (no error)"=w456, "Variant"=w465) -> ("error out"=w455:errorcluster, "Cluster Elements"=w464:variant[])  [unwired: 8 in]
                  n142 = Unbundle By Name(w454) -> ("Left"=w453:i16, "Bottom"=w452:i16)
                  n143 = for {
                    tunnel: w464 -> [w468] mode=indexing
                    tunnel: [w467] -> w463 mode=indexing
                    tunnel: [w466] -> w462 mode=indexing
                    n144 = call <vilib>:"GetTypeInfo.vi"("Variant"=w468) -> ("Name"=w466:string, "Type Enum"=w467:T17)  [unwired: 6 in, 3 out]
                  }
                  n145 = Equal?(x=i16 0, y=w453) -> (x = y?=w449:bool)
                  n146 = Equal?(x=w452, y=i16 32) -> (x = y?=w448:bool)
                  n147 = Equal?(x=w463, y=w460) -> (x = y?=w459:bool)
                  n148 = Equal?(x=w462, y=w461) -> (x = y?=w458:bool)
                  n149 = Compound Arithmetic op=AND(w459, w458, w449, w448) -> (w457:bool)
                }
                frame "LabVIEW Class Instance" {
                  n150 = call <vilib>:"GetLVClassInfo.vi"("error in (no error)"=w481, "Variant"=w482) -> ("error out"=w480:errorcluster, "Fully Qualified LV Class Name"=w478:string[])  [unwired: 7 in, 1 out]
                  n151 = Unbundle By Name(w472) -> ("Left"=w476:i16, "Top"=w475:i16)
                  n152 = Equal?(x=w479, y=w478) -> (x = y?=w477:bool)
                  n153 = Equal?(x=i16 0, y=w476) -> (x = y?=w470:bool)
                  n154 = Equal?(x=w475, y=i16 0) -> (x = y?=w469:bool)
                  n155 = Compound Arithmetic op=AND(w477, w470, w469) -> (w471:bool)
                }
              }
              n156 = Compound Arithmetic op=OR(w430, invert w410, w426) -> (w424:bool)
              n157 = case shown="False" w424 {
                tunnel: w415 -> [w436 w443]
                tunnel: w419 -> [w435 w442]
                tunnel: [w435 w441] -> w416
                tunnel: w418 -> [w438 w440]
                tunnel: [w437 w440] -> w417
                tunnel: w414 -> [w434 w439]
                tunnel: [w433 w439] -> w413
                tunnel: w412 -> [w432 _]
                frame False {
                  n158 = Build Array (concatenate)(w438, w436) -> (w437:refnum<vi>[])
                  n159 = Build Array (concatenate)(w434, w432) -> (w433:T16)
                }
                frame True {
                  n160 = Close Reference(reference=w443, error in (no error)=w442) -> (error out=w441:errorcluster)
                }
              }
            }
            frame True {
            }
          }
        }
        n161 = invoke class="Pnl" method="Make Selection"(reference=w362, error in=w360, "Objects"=w344) -> (reference out=w358:refnum<vi>, error out=w357:errorcluster)  [unwired: 1 in, 2 out]
        n162 = invoke class="Pnl" method="Copy Selection"(reference=w358, error in=w357) -> (reference out=w337:refnum<vi>, error out=w339:errorcluster)  [unwired: 1 in, 1 out]
        n163 = invoke class="Pnl" method="Clear Selection"(reference=w337, error in=w339) -> (reference out=w336:refnum<vi>, error out=w338:errorcluster)  [unwired: 1 in, 1 out]
        n164 = for {
          tunnel: w344 -> [w396] mode=indexing
          shift-right: [w392] -> w343
          shift-left: w338 -> [w393]
          tunnel: [w391] -> w342 mode=indexing
          n165 = property class="Ctl"(reference=w396, error in=w393) -> (error out=w392:errorcluster, "Label.Text"=w395:string, "Style"=w394:u32)  [unwired: 1 out]
          n166 = Bundle("Label.Text"=w395, "Style"=w394) -> (w391:cluster{"Label.Text":string, "Style":u32})  [unwired: 1 in]
        }
        n167 = Bundle By Name(cluster=w378, "Pattern"=w374, "Wiring Rules"=w377, "MemberDataTypes"=w342) -> (w376:T1)
        n168 = Close Reference(reference=w336, error in (no error)=w343) -> (error out=w383:errorcluster)
        n169 = Close Reference(reference=w344, error in (no error)=w383) -> (error out=w384:errorcluster)
        n170 = Close Reference(reference=w382, error in (no error)=w384) -> (error out=w379:errorcluster)
      }
      frame "AddMemberData" {
        (unwired) -1 ("index")
        w507 = refnum<vi> refnum  # Cluster
        n171 = Unbundle By Name(w489) -> ("MessageClassRef"=w486:refnum<vi>, "New Class Path"=w514:path, "Wiring Rules"=w502:T16, "MemberDataTypes"=w497:cluster{"Label.Text":string, "Style":u32}[])
        n172 = property class="LVClassLibrary"(reference=w486, error in=w503) -> (error out=w494:errorcluster, "Member Data"=w493:refnum<vi>)  [unwired: 1 out]
        n173 = Empty Array?(array=w502) -> (empty?=w501:bool)
        n174 = disable-structure shown="Enabled" {
          disable-tunnel: w494 -> [w520 w522]
          disable-tunnel: w493 -> [w519 w521]
          disable-tunnel: [w518 w522] -> w491
          disable-tunnel: [w517 w521] -> w492
          frame Enabled {
            n175 = invoke class="VI" method="FP.Open"(reference=w519, error in=w520, "Activate"=TRUE ("Activate?"), "State"=T2."Standard") -> (reference out=w517:refnum<vi>, error out=w518:errorcluster)  [unwired: 1 in, 3 out]
          }
          frame Disabled {
          }
        }
        n176 = property class="VI"(reference=w492, error in=w491) -> (reference out=w487:refnum<vi>, error out=w511:errorcluster, "Panel"=w513:refnum<vi>)
        n177 = property class="Pnl"(reference=w513, error in=w511) -> (reference out=w509:refnum<vi>, error out=w506:errorcluster, "Panes[]"=w512:refnum<vi>[], "Controls[]"=w510:refnum<vi>[])
        n178 = Index Array(array=w510) -> (element=w508:refnum<vi>)  [unwired: 1 in]
        n179 = To More Specific Class(target class=w507, reference=w508, error in=w506) -> (specific class reference=w505:refnum<vi>, error out=w504:errorcluster)
        n180 = property class="Clust"(reference=w505, error in=w504) -> (error out=w500:errorcluster, "Controls[]"=w499:refnum<vi>[])  [unwired: 1 out]
        n181 = for {
          shift-right: [w584] -> _
          shift-left: w500 -> [w588]
          tunnel: w499 -> [w587] mode=indexing
          tunnel: [w583] -> w498 mode=indexing
          n182 = property class="Ctl"(reference=w587, error in=w588) -> (error out=w584:errorcluster, "Label.Text"=w586:string, "Style"=w585:u32)  [unwired: 1 out]
          n183 = Bundle("Label.Text"=w586, "Style"=w585) -> (w583:cluster{"Label.Text":string, "Style":u32})  [unwired: 1 in]
        }
        n184 = Equal?(x=w497, y=w498) -> (x = y?=w496:bool)
        n185 = case shown="False" w496 {
          tunnel: w514 -> [w541 _]
          tunnel: w487 -> [w540 _]
          tunnel: [w524 w574] -> w490
          tunnel: w512 -> [w535 w577]
          tunnel: w509 -> [w533 w575]
          tunnel: w508 -> [w532 w580]
          tunnel: w501 -> [w530 _]
          tunnel: w500 -> [w528 w581]
          tunnel: w499 -> [w527 w582]
          tunnel: ["CreateSendMethod" "CloseRefs"] -> w495
          tunnel: w486 -> [w525 _]
          frame False {
            n186 = case shown="True" w530 {
              tunnel: w527 -> [w542 w546]
              tunnel: [w542 w544] -> w529
              frame False {
              }
              frame True {
                n187 = Delete From Array(array=w546, index=0) -> (deleted portion=w543:refnum<vi>, array with subset deleted=w544:refnum<vi>[])  [unwired: 1 in]
                n188 = Close Reference(reference=w543) -> ()  [unwired: 1 in, 1 out]
              }
            }
            n189 = for {
              tunnel: w529 -> [w572] mode=indexing
              shift-right: [w570] -> w531
              shift-left: w528 -> [w571]
              n190 = invoke class="Ctl" method="Delete"(reference=w572, error in=w571) -> (error out=w570:errorcluster)  [unwired: 1 in, 2 out]
            }
            n191 = Index Array(array=w535) -> (element=w534:refnum<vi>)  [unwired: 1 in]
            n192 = case shown="False" w530 {
              tunnel: [w560 w567] -> w539
              tunnel: w534 -> [w558 w569]
              tunnel: w533 -> [w550 _]
              tunnel: w532 -> [w552 _]
              tunnel: w531 -> [w551 w568]
              frame False {
                n193 = invoke class="Pane" method="Paste Selection"(reference=w558, error in=w551, "Pos"=T3 {"Left"=0, "Top"=0} ("Position")) -> (reference out=w556:refnum<vi>, error out=w557:errorcluster)  [unwired: 1 in, 2 out]
                n194 = Close Reference(reference=w556, error in (no error)=w557) -> (error out=w555:errorcluster)
                n195 = property class="Pnl"(reference=w550, error in=w555) -> (reference out=w548:refnum<vi>, error out=w553:errorcluster, "SelList[]"=w554:refnum<vi>[])
                n196 = for {
                  tunnel: w554 -> [w566] mode=indexing
                  shift-right: [w563] -> w549
                  shift-left: w553 -> [w564]
                  tunnel: w552 -> [w561]
                  n197 = invoke class="GObj" method="Move"(reference=w566, error in=w564, "position"=T3 {"Left"=0, "Top"=0}, "owner"=w561, "duplicate"=FALSE ("Duplicate? (F)")) -> (error out=w563:errorcluster)  [unwired: 1 in, 5 out]
                }
                n198 = invoke class="Pnl" method="Clear Selection"(reference=w548, error in=w549) -> (reference out=w547:refnum<vi>)  [unwired: 1 in, 2 out]
                n199 = Close Reference(reference=w547) -> (error out=w560:errorcluster)  [unwired: 1 in]
              }
              frame True {
                n200 = Close Reference(reference=w569, error in (no error)=w568) -> (error out=w567:errorcluster)
              }
            }
            n201 = invoke class="VI" method="CtlVIApplyChanges"(reference=w540, error in=w539) -> (reference out=w538:refnum<vi>, error out=w537:errorcluster)  [unwired: 1 in, 1 out]
            n202 = invoke class="VI" method="Save.Instrument"(reference=w538, error in=w537, "Path to saved file"=w541, "Save a Copy"=FALSE) -> (error out=w523:errorcluster)  [unwired: 2 in, 5 out]
            n203 = invoke class="LVClassLibrary" method="Save"(reference=w525, error in=w523) -> (error out=w524:errorcluster)  [unwired: 2 in, 3 out]
          }
          frame True {
            n204 = Close Reference(reference=w582, error in (no error)=w581) -> (error out=w579:errorcluster)
            n205 = Close Reference(reference=w580, error in (no error)=w579) -> (error out=w578:errorcluster)
            n206 = Close Reference(reference=w577, error in (no error)=w578) -> (error out=w576:errorcluster)
            n207 = Close Reference(reference=w575, error in (no error)=w576) -> (error out=w574:errorcluster)
          }
        }
        n208 = Bundle By Name(cluster=w489, "MemberData"=w487) -> (w488:T1)
      }
      frame "CreateSendMethod" {
        n209 = Unbundle By Name(w598) -> ("Update"=w591:bool, "New Class Path"=w599:path)  [unwired: 1 out]
        n210 = call <vilib>:"Get File Extension.vi"("file"=w590) -> ("filename without extension"=w589:string)  [unwired: 6 in, 4 out]
        n211 = Strip Path(path=w599) -> (stripped path=w594:path)  [unwired: 1 out]
        n212 = Format Into String(format string="Send %s.vi", w589) -> (resulting string=w592:string)  [unwired: 2 in, 1 out]
        n213 = Build Path(base path=w594, name or relative path=w592) -> (appended path=w596:path)
        n214 = case shown="False" w591 {
          tunnel: [w615 w616] -> w602
          tunnel: w601 -> [w614 w616]
          tunnel: w600 -> [w613 _]
          tunnel: w596 -> [w612 _]
          tunnel: w594 -> [w609 _]
          frame False {
            n215 = Build Path(base path=w609, name or relative path="Send Template.vi") -> (appended path=w606:path)
            n216 = Open VI Reference(application reference (local)=w613, vi path=w606, error in (no error)=w614) -> (vi reference=w611:refnum<vi>, error out=w607:errorcluster)  [unwired: 3 in]
            n217 = invoke class="VI" method="Save.Instrument"(reference=w611, error in=w607, "Path to saved file"=w612, "Save a Copy"=FALSE) -> (reference out=w610:refnum<vi>, error out=w603:errorcluster)  [unwired: 2 in, 4 out]
            n218 = Close Reference(reference=w610, error in (no error)=w603) -> (error out=w605:errorcluster)
            n219 = Delete(path (use dialog)=w606, error in=w605) -> (error out=w615:errorcluster)  [unwired: 3 in, 2 out]
          }
          frame True {
          }
        }
        n220 = Bundle By Name(cluster=w598, "New Send Method"=w596) -> (w597:T1)
      }
      frame "BuildSendMethod" {
        n221 = Unbundle By Name(w661) -> ("MemberData"=w620:refnum<vi>, "MessageClassRef"=w621:refnum<vi>, "New Send Method"=w653:path, "Wiring Rules"=w652:T16, "Update"=w628:bool)
        n222 = Unbundle By Name(w661) -> ("Pattern"=w635:u32)
        n223 = Open VI Reference(application reference (local)=w663, vi path=w653, error in (no error)=w665) -> (vi reference=w625:refnum<vi>, error out=w624:errorcluster)  [unwired: 3 in]
        n224 = disable-structure shown="Enabled" {
          disable-tunnel: w624 -> [w673 w675]
          disable-tunnel: w625 -> [w672 w674]
          disable-tunnel: [w671 w675] -> w622
          disable-tunnel: [w670 w674] -> w623
          frame Disabled {
            n225 = invoke class="VI" method="FP.Open"(reference=w672, error in=w673, "Activate"=TRUE ("Activate?"), "State"=T2."Standard") -> (reference out=w670:refnum<vi>, error out=w671:errorcluster)  [unwired: 1 in, 3 out]
          }
          frame Enabled {
          }
        }
        n226 = case shown="True" w628 {
          tunnel: w623 -> [w676 w680]
          tunnel: w622 -> [w677 w681]
          tunnel: [w677 w678] -> w627
          tunnel: [w676 w679] -> w626
          frame False {
          }
          frame True {
            n227 = call <resource>:"MM_RemoveControls.vi"("error in (no error)"=w681, "vi ref in"=w680) -> ("error out"=w678:errorcluster, "vi ref out"=w679:refnum<vi>)  [unwired: 8 in]
          }
        }
        n228 = property class="VI"(reference=w626, error in=w627) -> (error out=w639:errorcluster, "ConPane"=w640:refnum<vi>)  [unwired: 1 out]
        n229 = property class="ConPane"(reference=w640, error in=w639, "Pattern"=w635) -> (reference out=w636:refnum<vi>, error out=w638:errorcluster)
        n230 = Close Reference(reference=w636, error in (no error)=w638) -> (error out=w637:errorcluster)
        n231 = call <resource>:"MM_PasteControls.vi"("Position"=T3 {"Left"=396, "Top"=0}, "error in (no error)"=w637, "vi ref in"=w626) -> ("error out"=w632:errorcluster, "Controls"=w667:refnum<vi>[], "vi ref out"=w634:refnum<vi>)  [unwired: 6 in]
        n232 = Array Size(array=w667) -> (size(s)=w658:i32)
        n233 = property class="LVClassLibrary"(reference=w621, error in=w632) -> (error out=w633:errorcluster, "Path"=w642:path)  [unwired: 1 out]
        n234 = call <vilib>:"TRef Traverse for References.vi"("Traverse Target"=TRef_TravTarget."BD", "error in (no error)"=w633, "Class Name"="LabVIEWClassConstant", "VI Refnum"=w634) -> ("error out"=w647:errorcluster, "References"=w651:refnum<vi>[], "dup VI Refnum"=w643:refnum<vi>)  [unwired: 4 in, 1 out]
        n235 = Index Array(array=w651) -> (element=w650:refnum<vi>)  [unwired: 1 in]
        n236 = invoke class="GObj" method="Replace"(reference=w650, error in=w647, "Path"=w642) -> (error out=w649:errorcluster, "Replace"=w648:refnum<vi>)  [unwired: 3 in, 4 out]
        n237 = Close Reference(reference=w648, error in (no error)=w649) -> (error out=w644:errorcluster)
        n238 = case shown="1, Default" w658 {
          tunnel: [w684 w702] -> w655
          tunnel: [w683 w701] -> w656
          tunnel: w644 -> [w687 w700]
          tunnel: w643 -> [w686 w699]
          tunnel: w667 -> [_ w698]
          tunnel: w652 -> [_ w695]
          tunnel: w620 -> [_ w694]
          frame 0 {
            n239 = disable-structure shown="Enabled" {
              disable-tunnel: w687 -> [w691 w693]
              disable-tunnel: w686 -> [w690 w692]
              disable-tunnel: [w689 w693] -> w685
              disable-tunnel: [w688 w692] -> w682
              frame Disabled {
                n240 = call <resource>:"MM_WireClass.vi"("error in (no error)"=w691, "vi reference"=w690) -> ("error out"=w689:errorcluster, "dup VI Refnum"=w688:refnum<vi>)  [unwired: 8 in]
              }
              frame Enabled {
              }
            }
            n241 = invoke class="VI" method="BD.Remove Bad Wires"(reference=w682, error in=w685) -> (reference out=w683:refnum<vi>, error out=w684:errorcluster)  [unwired: 1 in, 1 out]
          }
          frame 1, Default {
            # "Fix to support more terminals"
            n242 = call <resource>:"MM_ConnectControlsToCP.vi"("error in (no error)"=w700, "Wiring Rules"=w695, "Controls"=w698, "vi ref in"=w699) -> ("error out"=w697:errorcluster, "vi ref out"=w696:refnum<vi>)  [unwired: 6 in]
            n243 = call <resource>:"MM_WireControlsToBundler.vi"("MessageClassRef"=w694, "error in (no error)"=w697, "Controls"=w698, "vi reference in"=w696) -> ("error out"=w702:errorcluster, "vi reference out"=w701:refnum<vi>)  [unwired: 6 in]
          }
        }
        n244 = invoke class="VI" method="BD.CleanUp"(reference=w656, error in=w655) -> (reference out=w619:refnum<vi>, error out=w641:errorcluster)  [unwired: 1 in, 1 out]
        n245 = property class="VI"(reference=w619, error in=w641) -> (reference out=w630:refnum<vi>, error out=w629:errorcluster, "ConPane"=w631:refnum<vi>)
        n246 = call <resource>:"MM_CleanUpPanel.vi"("error in (no error)"=w629, "Conpane"=w631, "VI Refnum"=w630) -> ("error out"=w617:errorcluster)  [unwired: 8 in]
        n247 = call <vilib>:"Apply New VI Tools-Options Settings.vi"("error in (no error)"=w617, "VI Refnum"=w619) -> ("dup VI Refnum"=w618:refnum<vi>)  [unwired: 8 in, 1 out]
        n248 = invoke class="VI" method="Save.Instrument"(reference=w618, error in=w617, "Path to saved file"=w653, "Save a Copy"=FALSE) -> (reference out=w660:refnum<vi>, error out=w659:errorcluster)  [unwired: 2 in, 4 out]
        n249 = Close Reference(reference=w660, error in (no error)=w659) -> (error out=w666:errorcluster)
        n250 = Close Reference(reference=w667, error in (no error)=w666) -> (error out=w664:errorcluster)
      }
      frame "BuildDo" {
        n251 = Unbundle By Name(w708) -> ("Class Name"=w712:string, "Target Actor Method path"=w738:path, "Update"=w713:bool, "Destination Path"=w705:path)
        n252 = Unbundle By Name(w708) -> ("ActorClassPath"=w707:path)
        n253 = Build Path(base path=w705, name or relative path="Do.vi") -> (appended path=w704:path)
        n254 = Open VI Reference(application reference (local)=w740, vi path=w704, error in (no error)=w739) -> (vi reference=w735:refnum<vi>, error out=w736:errorcluster)  [unwired: 3 in]
        n255 = disable-structure shown="Enabled" {
          disable-tunnel: w736 -> [w807 w809]
          disable-tunnel: w735 -> [w806 w808]
          disable-tunnel: [w805 w809] -> w731
          disable-tunnel: [w804 w808] -> w730
          frame Disabled {
            n256 = invoke class="VI" method="FP.Open"(reference=w806, error in=w807, "Activate"=TRUE ("Activate?"), "State"=T2."Standard") -> (reference out=w804:refnum<vi>, error out=w805:errorcluster)  [unwired: 1 in, 3 out]
          }
          frame Enabled {
          }
        }
        n257 = case shown="True" w713 {
          tunnel: w738 -> [w756 _]
          tunnel: w707 -> [w755 _]
          tunnel: w731 -> [w749 w784]
          tunnel: w730 -> [w748 w780]
          tunnel: "LabVIEWClassConstant" ("Class Name") -> [w747 _]
          tunnel: TRef_TravTarget."BD" ("Traverse Target") -> [w744 w775]
          tunnel: [w743 w778] -> w727
          tunnel: [w742 w777] -> w726
          tunnel: ["UpdateIcons" "CloseRefs"] -> w711
          frame False {
            n258 = call <vilib>:"TRef Traverse for References.vi"("Traverse Target"=w744, "error in (no error)"=w749, "Class Name"=w747, "VI Refnum"=w748) -> ("error out"=w750:errorcluster, "References"=w754:refnum<vi>[], "dup VI Refnum"=w745:refnum<vi>)  [unwired: 4 in, 1 out]
            n259 = Index Array(array=w754) -> (element=w753:refnum<vi>)  [unwired: 1 in]
            n260 = invoke class="GObj" method="Replace"(reference=w753, error in=w750, "Path"=w755) -> (error out=w752:errorcluster, "Replace"=w751:refnum<vi>)  [unwired: 3 in, 4 out]
            n261 = Close Reference(reference=w751, error in (no error)=w752) -> (error out=w746:errorcluster)
            n262 = while {
              tunnel: w746 -> [w772]
              tunnel: w745 -> [w771]
              tunnel: w756 -> [w770]
              tunnel: w744 -> [w768]
              tunnel: [w761] -> w743
              tunnel: [w767] -> w742
              stop <- w762 stop-if-true
              n263 = call <vilib>:"TRef Traverse for References.vi"("Traverse Target"=w768, "error in (no error)"=w772, "Class Name"="SubVI" ("GObj Class Name"), "VI Refnum"=w771) -> ("error out"=w773:errorcluster, "References"=w760:refnum<vi>[], "dup VI Refnum"=w767:refnum<vi>)  [unwired: 4 in, 1 out]
              n264 = Delete From Array(array=w760, index=0) -> (deleted portion=w757:refnum<vi>, array with subset deleted=w758:refnum<vi>[])  [unwired: 1 in]
              n265 = invoke class="GObj" method="Replace"(reference=w757, error in=w773, "Path"=w770) -> (error out=w765:errorcluster, "Replace"=w764:refnum<vi>)  [unwired: 3 in, 4 out]
              n266 = Close Reference(reference=w758) -> ()  [unwired: 1 in, 1 out]
              n267 = call <resource>:"MM_RewireDo.vi"("error in (no error)"=w765, "Replace"=w764) -> ("error out"=w761:errorcluster, "done?"=w763:bool)  [unwired: 8 in]
              n268 = Unbundle By Name(w761) -> ("status"=w766:bool)
              n269 = Or(x=w763, y=w766) -> (x .or. y?=w762:bool)
            }
          }
          frame True {
            n270 = call <vilib>:"TRef Traverse for References.vi"("Traverse Target"=w775, "error in (no error)"=w784, "Class Name"="Unbundler", "VI Refnum"=w780) -> ("error out"=w791:errorcluster, "References"=w787:refnum<vi>[])  [unwired: 4 in, 2 out]
            n271 = Index Array(array=w787) -> (element=w790:refnum<vi>)  [unwired: 1 in]
            n272 = To More Specific Class(target class=refnum<vi> refnum ("reference"), reference=w790, error in=w791) -> (specific class reference=w786:refnum<vi>, error out=w785:errorcluster)
            n273 = property class="Unbundler"(reference=w786, error in=w785) -> (reference out=w781:refnum<vi>, error out=w783:errorcluster, "OutputTerms[]"=w782:refnum<vi>[])
            n274 = for {
              tunnel: w782 -> [w797] mode=indexing
              shift-right: [w794] -> w774
              shift-left: w783 -> [w796]
              n275 = property class="Term"(reference=w797, error in=w796) -> (error out=w795:errorcluster, "Wire"=w793:refnum<vi>)  [unwired: 1 out]
              n276 = Not A Number/Path/Refnum?(number/path/refnum=w793) -> (NaN/Path/Refnum?=w792:bool)
              n277 = case shown="False" w792 {
                tunnel: w795 -> [w800 w801]
                tunnel: [w799 w801] -> w794
                tunnel: w793 -> [w798 _]
                frame False {
                  n278 = invoke class="Wire" method="Delete"(reference=w798, error in=w800) -> (error out=w799:errorcluster)  [unwired: 1 in, 2 out]
                }
                frame True {
                }
              }
            }
            n279 = Close Reference(reference=w782, error in (no error)=w774) -> ()  [unwired: 1 out]
            n280 = Close Reference(reference=w781, error in (no error)=w774) -> (error out=w779:errorcluster)
            n281 = invoke class="VI" method="BD.Remove Bad Wires"(reference=w780, error in=w779) -> (reference out=w777:refnum<vi>, error out=w778:errorcluster)  [unwired: 1 in, 1 out]
          }
        }
        n282 = call <resource>:"MM_WireFPControlsToUnBundler.vi"("error in (no error)"=w727, "vi reference in"=w726) -> ("error out"=w717:errorcluster, "vi reference out"=w716:refnum<vi>)  [unwired: 8 in]
        n283 = property class="VI"(reference=w716, error in=w717) -> (reference out=w714:refnum<vi>, error out=w720:errorcluster, "Panel"=w718:refnum<vi>)
        n284 = property class="Pnl"(reference=w718, error in=w720) -> (reference out=w725:refnum<vi>, error out=w721:errorcluster, "Controls[]"=w719:refnum<vi>[])
        n285 = for {
          tunnel: w719 -> [w817] mode=indexing
          shift-right: [w812] -> w722
          shift-left: w721 -> [w814]
          tunnel: [w811] -> w723 mode=indexing
          tunnel: w712 -> [w810]
          n286 = property class="Ctl"(reference=w817, error in=w814) -> (reference out=w815:refnum<vi>, error out=w813:errorcluster, "Label.Text"=w816:string)
          n287 = case shown="Default" w816 {
            tunnel: w815 -> [w818 w824]
            tunnel: w813 -> [w819 w823]
            tunnel: [w819 w822] -> w812
            tunnel: [w818 w821] -> w811
            tunnel: w810 -> [_ w820]
            frame Default {
            }
            frame "Message Template" {
              n288 = property class="Ctl"(reference=w824, error in=w823, "Label.Text"=w820) -> (reference out=w821:refnum<vi>, error out=w822:errorcluster)
            }
          }
        }
        n289 = Close Reference(reference=w723, error in (no error)=w722) -> (error out=w724:errorcluster)
        n290 = Close Reference(reference=w725, error in (no error)=w724) -> (error out=w715:errorcluster)
        n291 = invoke class="VI" method="BD.CleanUp"(reference=w714, error in=w715) -> (reference out=w710:refnum<vi>, error out=w703:errorcluster)  [unwired: 1 in, 1 out]
        n292 = call <vilib>:"Apply New VI Tools-Options Settings.vi"("error in (no error)"=w703, "VI Refnum"=w710) -> ("dup VI Refnum"=w709:refnum<vi>)  [unwired: 8 in, 1 out]
        n293 = invoke class="VI" method="Save.Instrument"(reference=w709, error in=w703, "Path to saved file"=w704, "Save a Copy"=FALSE) -> (reference out=w734:refnum<vi>, error out=w733:errorcluster)  [unwired: 2 in, 4 out]
        n294 = Close Reference(reference=w734, error in (no error)=w733) -> (error out=w737:errorcluster)
      }
      frame "UpdateIcons" {
        n295 = Unbundle By Name(w837) -> ("Version"=w832:string, "MessageClassRef"=w836:refnum<vi>, "ActorClassRef"=w830:refnum<vi>, "Update"=w828:bool, "ActorClassPath"=w825:path)
        n296 = call <vilib>:"Get File Extension.vi"("file"=w827) -> ("filename without extension"=w826:string)  [unwired: 6 in, 4 out]
        n297 = call <vilib>:"Get File Extension.vi"("file"=w834) -> ("filename without extension"=w833:string)  [unwired: 6 in, 4 out]
        n298 = call <vilib>:"Get File Extension.vi"("file"=w825) -> ("filename without extension"=w829:string)  [unwired: 6 in, 4 out]
        n299 = case shown="False" w828 {
          tunnel: w836 -> [w864 _]
          tunnel: [w863 w871] -> w835
          tunnel: w833 -> [w859 _]
          tunnel: w832 -> [w856 _]
          tunnel: w831 -> [w855 w871]
          tunnel: w830 -> [w853 _]
          tunnel: w829 -> [w849 _]
          tunnel: w826 -> [w845 _]
          frame False {
            n300 = call <resource>:"GDSLvClass_ReadClassType.vi"("Class Refnum In"=w853, "error in (no error)"=w855) -> ("ClassSettings"=w852:T6, "error out"=w854:errorcluster)  [unwired: 15 in, 1 out]
            n301 = Unbundle By Name(w852) -> ("ConnectorPanePattern"=w851:string)
            n302 = Bundle By Name(cluster=T9 {"LibraryIcon"="Normal", "HeaderRows(1)"=0} ("LibraryIcon"), "LibraryIcon"="Message", "HeaderRows(1)"=u8 3) -> (w869:T9)
            n303 = call <resource>:"GDSLvIcon_DialogUpdateClass.vi"("ClassPath(FilePath/ProjectTreePath/LvCLassRef)"=w864, "ClassName"=w845, "AutoUpdate"=TRUE, "error in (no error)"=w854, "LibraryIcon"=w869) -> ("error out"=w843:errorcluster)  [unwired: 11 in, 3 out]
            n304 = Format Into String(format string="Message class for Actor: %s", w849) -> (resulting string=w848:string)  [unwired: 2 in, 1 out]
            n305 = call <resource>:"AF_ConfigurationMemory.vi"("error in (no error)"=w843, "Action"=enum16{"Read", "Load", "Save", "Set"}."Read") -> ("AF_MessaageWireConfigurationOut"=w842:T13, "IconOut"=w841:string, "error out"=w840:errorcluster)  [unwired: 14 in, 1 out]
            n306 = call <resource>:"GOOP_WirePenTranslator.vi"("WireConfigurationIn"=w842) -> ("WirePensOut"=w865:T15)  [unwired: 17 in, 1 out]
            n307 = call <resource>:"GDSLvClass_StoreClassItemIcon.vi"("Library Refnum"=w864, "ClassItemIconName"=w841, "error in (no error)"=w840) -> ("error out"=w866:errorcluster)  [unwired: 15 in, 1 out]
            n308 = property class="LVClassLibrary"(reference=w864, error in=w866, "Wire Pens"=w865) -> (reference out=w847:refnum<vi>, error out=w860:errorcluster)
            n309 = Format Into String(LvNativeProviderName."Endevo LabVIEW Native" ("ProviderName")) -> (resulting string=w857:string)  [unwired: 3 in, 1 out]
            n310 = Bundle By Name(cluster=T6 {"ClassProviderName"="", "ClassTemplateUsed"="", "ClassTemplateVersion"="", "ClassDescription"="", "PlugIns"=[], "ConnectorPanePattern"=""} ("ClassSettings"), "ClassProviderName"=w857, "ClassTemplateUsed"=w859, "ClassTemplateVersion"=w856, "ClassDescription"=w848, "ConnectorPanePattern"=w851) -> (w862:T6)
            n311 = call <resource>:"GDSLvClass_StoreClassType.vi"("Class Refnum In"=w847, "ClassSettings"=w862, "error in (no error)"=w860) -> ("error out"=w839:errorcluster)  [unwired: 15 in, 1 out]
            n312 = invoke class="LVClassLibrary" method="Save"(reference=w847, error in=w839) -> (error out=w863:errorcluster)  [unwired: 2 in, 3 out]
          }
          frame True {
          }
        }
      }
      frame "AddToProject" {
        n313 = Unbundle By Name(w876) -> ("MessageClassRef"=w897:refnum<vi>, "New Class Path"=w877:path, "ActorClassRef"=w896:refnum<vi>, "Destination Path"=w887:path, "ActorClassParentItem"=w885:refnum<vi>)
        n314 = Strip Path(path=w887) -> (stripped path=w886:path)  [unwired: 1 out]
        n315 = property class="LVClassLibrary"(reference=w897, error in=w903) -> (error out=w873:errorcluster, "Name"=w879:string, "Type String"=w878:string)  [unwired: 1 out]
        n316 = call <resource>:"AF_ConfigurationMemory.vi"("error in (no error)"=w873, "Action"=enum16{"Read", "Load", "Save", "Set"}."Read") -> ("AF_SettingsOut"=w891:T11, "error out"=w872:errorcluster)  [unwired: 14 in, 2 out]
        n317 = Unbundle By Name(w891) -> ("MessageFolderName"=w888:string)
        n318 = property class="LVClassLibrary"(reference=w896, error in=w872) -> ("Parent"=w893:refnum<vi>)  [unwired: 2 out]
        n319 = Build Array (concatenate)(w888, string[] ["Message", "Messages", "Msg"] ("1D array")) -> (w889:string[])
        n320 = To Lower Case(string=w889) -> (all lower case string=w901:string[])
        n321 = property class="ProjectItem"(reference=w893) -> ("Children[]"=w895:refnum<vi>[])  [unwired: 1 in, 2 out]
        n322 = for {
          tunnel: w895 -> [w964] mode=indexing
          tunnel: w901 -> [w955]
          tunnel: [w958] -> w900
          tunnel: [w957] -> w899
          stop <- w957 stop-if-true
          n323 = property class="ProjectItem"(reference=w964) -> (reference out=w958:refnum<vi>, "Name"=w963:string, "Type String"=w962:string)  [unwired: 1 in, 1 out]
          n324 = To Lower Case(string=w963) -> (all lower case string=w956:string)
          n325 = for {
            tunnel: w956 -> [w968]
            tunnel: w955 -> [w967] mode=indexing
            tunnel: [w965] -> w954
            stop <- w965 stop-if-true
            n326 = Match Pattern(string=w968, regular expression=w967) -> (offset past match=w966:i32)  [unwired: 1 in, 3 out]
            n327 = Greater Or Equal To 0?(x=w966) -> (x >= 0?=w965:bool)
          }
          n328 = To Lower Case(string=w962) -> (all lower case string=w961:string)
          n329 = Equal?(x=w961, y="folder") -> (x = y?=w959:bool)
          n330 = And(x=w959, y=w954) -> (x .and. y?=w957:bool)
        }
        n331 = case shown="False" w899 {
          tunnel: [w934 w938] -> w883
          tunnel: w893 -> [_ w937]
          tunnel: w900 -> [w934 _]
          tunnel: w888 -> [_ w936]
          tunnel: w886 -> [_ _]
          tunnel: w885 -> [_ w935]
          frame True {
          }
          frame False {
            n332 = To More Specific Class(target class=refnum<vi> refnum ("reference"), reference=w937) -> (specific class reference=w939:refnum<vi>, error out=w940:errorcluster)  [unwired: 1 in]
            n333 = case shown="No Error" w940 {
              tunnel: w939 -> [w946 _]
              tunnel: [w944 w949] -> w938
              tunnel: w937 -> [_ _]
              tunnel: w936 -> [w942 w951]
              tunnel: w935 -> [_ w950]
              frame No Error {
                n334 = invoke class="Library" method="AddItem"(reference=w946, "Name"=w942, "Path"=path "", "Type"="Folder") -> ("AddItem"=w944:refnum<vi>)  [unwired: 2 in, 5 out]
              }
              frame Error {
                n335 = invoke class="ProjectItem" method="AddItem"(reference=w950, "Name"=w951, "Path"=path "", "Type"="Folder") -> (error out=w947:errorcluster, "AddItem"=w948:refnum<vi>)  [unwired: 2 in, 4 out]
                n336 = Select(t=w950, s=w947, f=w948) -> (s? t:f=w949:refnum<vi>)
              }
            }
          }
        }
        n337 = Not A Number/Path/Refnum?(number/path/refnum=w883) -> (NaN/Path/Refnum?=w884:bool)
        n338 = property class="ProjectItem"(reference=w883) -> ("Name"=w881:string, "Type String"=w880:string)  [unwired: 1 in, 2 out]
        n339 = Format Into String(format string="PI:%s(%s):Add:%s(%s:%s)", w881, w880, w879, w878, w877) -> (resulting string=w874:string)  [unwired: 2 in, 1 out]
        n340 = case shown="False" w884 {
          tunnel: w879 -> [w916 _]
          tunnel: w878 -> [w915 _]
          tunnel: w877 -> [w911 _]
          tunnel: [w909 w933] -> w898
          tunnel: w873 -> [w908 w932]
          tunnel: w897 -> [w907 w933]
          tunnel: [w906 w932] -> w894
          tunnel: w883 -> [w905 _]
          tunnel: w874 -> [_ _]
          frame False {
            n341 = invoke class="ProjectItem" method="AddItem"(reference=w905, error in=w908, "Name"=w916, "Path"=w911, "Type"=w915) -> (reference out=w914:refnum<vi>, error out=w913:errorcluster, "AddItem"=w912:refnum<vi>)  [unwired: 1 in, 3 out]
            n342 = case shown="Error" w913 {
              selector: w913 -> [w921 w928]
              tunnel: w908 -> [_ w929]
              tunnel: [w918 w927] -> w910
              tunnel: w912 -> [w924 _]
              tunnel: [w919 w925] -> w909
              tunnel: w907 -> [w917 w925]
              frame No Error {
                n343 = To More Specific Class(target class=refnum<vi> refnum ("reference"), reference=w924, error in=w921) -> (specific class reference=w923:refnum<vi>, error out=w920:errorcluster)
                n344 = invoke class="LVClassLibrary" method="Save"(reference=w923, error in=w920) -> (reference out=w919:refnum<vi>, error out=w918:errorcluster)  [unwired: 2 in, 2 out]
                n345 = Close Reference(reference=w917, error in (no error)=w918) -> ()  [unwired: 1 out]
              }
              frame Error {
                # "ignore error for autopopulating folders"
                n346 = Unbundle By Name(w928) -> ("code"=w931:i32)
                n347 = Equal?(x=w931, y=56002) -> (x = y?=w926:bool)
                n348 = Select(t=w929, s=w926, f=w928) -> (s? t:f=w927:errorcluster)
              }
            }
            n349 = Close Reference(reference=w914, error in (no error)=w910) -> (error out=w906:errorcluster)
          }
          frame True {
          }
        }
        n350 = Bundle By Name(cluster=w876, "DebugInfo"=w874) -> (w875:T1)
        n351 = Bundle By Name(cluster=w875, "MessageClassRef"=w898) -> (w902:T1)
        n352 = Close Reference(reference=w893, error in (no error)=w894) -> ()  [unwired: 1 out]
        n353 = Close Reference(reference=w895, error in (no error)=w894) -> ()  [unwired: 1 out]
      }
      frame "CloseRefs", "Error", Default {
        n354 = Unbundle By Name(w970) -> ("MemberData"=w979:refnum<vi>, "ActorClassRef"=w985:refnum<vi>, "MessageClassRef"=w982:refnum<vi>, "ActorClassParentItem"=w974:refnum<vi>)
        n355 = invoke class="App" method="Clipboard.Empty"(reference=w980) -> ()  [unwired: 2 in, 3 out]
        n356 = property class="VI"(reference=w979, "Front Panel.Open"=FALSE ("Front Panel Window:Open")) -> (reference out=w976:refnum<vi>, error out=w977:errorcluster)  [unwired: 1 in]
        n357 = Not A Number/Path/Refnum?(number/path/refnum=w982) -> (NaN/Path/Refnum?=w981:bool)
        n358 = Close Reference(reference=w976, error in (no error)=w977) -> (error out=w975:errorcluster)
        n359 = case shown="False" w981 {
          tunnel: [w994 w1013] -> w984
          tunnel: w983 -> [w990 w1013]
          tunnel: w982 -> [w989 _]
          tunnel: w975 -> [_ _]
          frame False {
            n360 = stacked-sequence {
              tunnel: w990 -> [w1002]
              tunnel: w989 -> [w1003]
              tunnel: [w1002] -> w988
              frame #0 {
                n361 = call <vilib>:"Apply New Library Tools-Options Settings.vi"("error in (no error)"=w1002, "Library Refnum"=w1003) -> ()  [unwired: 8 in, 2 out]
              }
            }
            n362 = call <resource>:"GDSLvClass_SaveEverythingInClass.vi"("ClassRefIn"=w989, "ForceResaving(False)"=TRUE, "error in"=w988) -> ("ClassRefOut"=w992:refnum<vi>, "error out"=w993:errorcluster)  [unwired: 15 in]
            n363 = property class="LVClassLibrary"(reference=w992, error in=w993) -> (reference out=w998:refnum<vi>, error out=w997:errorcluster, "Parent"=w987:refnum<vi>)
            n364 = To More Specific Class(target class=refnum<vi> refnum ("reference out"), reference=w987, error in=w997) -> (specific class reference=w999:refnum<vi>, error out=w1000:errorcluster)
            n365 = case shown="Error" w1000 {
              selector: w1000 -> [w1008 _]
              tunnel: w999 -> [w1009 _]
              tunnel: w998 -> [w1007 w1012]
              tunnel: w997 -> [_ w1011]
              tunnel: [w1007 w1012] -> w996
              tunnel: [w1004 w1011] -> w995
              tunnel: w987 -> [_ w1010]
              frame No Error {
                n366 = invoke class="Library" method="Save"(reference=w1009, error in=w1008) -> (reference out=w1006:refnum<vi>, error out=w1005:errorcluster)  [unwired: 2 in, 2 out]
                n367 = Close Reference(reference=w1006, error in (no error)=w1005) -> (error out=w1004:errorcluster)
              }
              frame Error {
                n368 = Close Reference(reference=w1010) -> ()  [unwired: 1 in, 1 out]
              }
            }
            n369 = Close Reference(reference=w996, error in (no error)=w995) -> (error out=w994:errorcluster)
          }
          frame True {
          }
        }
        n370 = Close Reference(reference=w985, error in (no error)=w984) -> (error out=w973:errorcluster)
        n371 = Close Reference(reference=w974, error in (no error)=w973) -> ()  [unwired: 1 out]
        n372 = Unbundle By Name(w970) -> ("DebugInfo"=w969:string)
        n373 = call <resource>:"GDSError_LogErrorInformation.vi"("State"=w971, "LocalVariableData"=w970, "ExtraErrorInfo"=w969, "error in (no error)"=w973) -> ("error out"=w972:errorcluster)  [unwired: 15 in]
      }
    }
    n374 = Equal?(x=w33, y="Exit") -> (x = y?=w36:bool)
    n375 = Select(t="Error", s=w25, f=w33) -> (s? t:f=w37:string)
  }
  "error out" <- w12
  n376 = disable-structure shown="Disabled" {
    disable-tunnel: _ -> [w1017 _]
    disable-tunnel: [w1015 _] -> _
    disable-tunnel: _ -> [w1014 _]
    frame Disabled {
      n377 = property class="App"(reference=w1017) -> ("App.AllMyLibses"=w1016:string[])  [unwired: 1 in, 2 out]
      n378 = while {
        tunnel: w1014 -> [w1022]
        shift-right: [w1019] -> w1015
        shift-left: w1014 -> [w1021]
        tunnel: w1016 -> [w1024]
        i -> [w1020]
        stop <- w1018 stop-if-true
        # "This loop ensures new msg name is not already used."
        n379 = Concatenate Strings(w1021, ".lvclass" ("string")) -> (w1025:string)
        n380 = Search 1D Array(1D array=w1024, element=w1025) -> (index of element=w1023:i32)  [unwired: 1 in]
        n381 = case shown="..-1" w1023 {
          tunnel: w1022 -> [_ w1035]
          tunnel: w1021 -> [w1028 _]
          tunnel: w1020 -> [_ w1033]
          tunnel: [w1028 w1029] -> w1019
          tunnel: [TRUE _] -> w1018
          frame ..-1 {
            # "Name is unique."
          }
          frame Default {
            n382 = call <vilib>:"Space Constant.vi"() -> ("String"=w1034:string)
            n383 = Add(x=w1033, y=2) -> (x+y=w1031:i32)
            n384 = Number To Decimal String(number=w1031) -> (decimal integer string=w1030:string)  [unwired: 1 in]
            n385 = Concatenate Strings(w1035, w1034, w1030) -> (w1029:string)
          }
        }
      }
    }
    frame Enabled {
    }
  }
